vi "slow_control_2_14.vi"() -> ()   [LabVIEW 2018]
uses:
  4623b864-5764-45c6-9cb2-3e18237880ca.vi
  fa57f61f-0bb9-49ac-92eb-fcb40add4dbb.vi
  499f9cf5-7b15-41ea-951a-8da9be12721d.vi
  <vilib>/DAQmx/read.llb/DAQmx Read (Analog 1D DBL NChan 1Samp).vi
  ffb0d1b3-ef19-4e2e-b36e-7277177ef4b3.vi
  9a1acc8a-69db-4048-9e4c-bb07d66d2422.vi
  <vilib>/DAQmx/create/channels.llb/DAQmx Create Channel (AI-Voltage-Basic).vi
  <vilib>/DAQmx/create/channels.llb/DAQmx Create Channel (AI-Current-Basic).vi
  <vilib>/DAQmx/create/channels.llb/DAQmx Create Channel (AI-Temperature-RTD).vi
  <vilib>/DAQmx/miscellaneous.llb/DAQmx Fill In Error Info.vi
  <vilib>/Utility/file.llb/Read Delimited Spreadsheet (string).vi
  <instrlib>/Lake Shore 335/Lake Shore 335.lvlib
  <instrlib>/CAEN PSM/CAEN PSM.lvlib
  <resource>/objmgr/daqmx.rc
panel:
  out "Heater":dbl
  out "Coldhead":dbl
  out "Cycle number":i32
  out "Alarm state":bool
  out "Timestamp last \nmeasured (UPS)":timestamp
  out "Auto-clear":bool
  in  "Auto-clear data?":bool
  in  "Clear data":bool
  in  "Clear data every N cycles":dbl
  in  "N samples":i32=30
  out "Average Flow (SLPM)":dbl caption="Flow (SLPM)"
  out "CAEN Ch. Names":string[](array[string])
  in  "Cycles to execute":dbl=5.0 format="%#_13g"
  out "Detector Pressure":dbl
  in  "N samples":i32=20
  in  "Allows tabs on \nfront panel":T1(tab)
  in  "Specify up to six temperature sensors inside \nthe detector, separated with a comma.\nNumbers only, single commas!":string="10,11,12,13,14,15"
  out "Valid example:":string="11,12, 13, 15 ,14 "
  in  "Anode ch.":enum16{"1", "2", "3", "4"}(ring)=enum."3"
  in  "CAEN unit selector":enum16{"CAEN 1", "CAEN 2"}(ring)
  in  "Multipliers":dbl[](array[numeric])=[1.0, 1.0, 1.0, 1.0, 1.0, 1.0, 1.0, 1.0]
  in  "Offsets\nsubtracted":dbl[](array[numeric])=[0.0, 0.0, 0.0, 0.0, 0.0, 0.0, 0.0, 0.0]
  in  "Channel Names (9207, ai8:15)":string[](array[string])=["i0", "i1", "i2", "i3", "i4", "i5", "i6", "i7"] caption="\"Other\""
  in  "Flow meter input:":u16(ring)=3 items=["v0", "v1", "v2", "v3", "v4", "v5", "v6", "v7"]
  in  "Detector pressure input:":u16(ring) items=["v0", "v1", "v2", "v3", "v4", "v5", "v6", "v7"]
  in  "Channel Names (9207, ai0:7)":string[](array[string])=["v0", "v1", "v2", "v3", "v4", "v5", "v6", "v7"] caption="\"Other\""
  in  "Multipliers":dbl[](array[numeric])=[1.0, 1.0, 1.0, 1.0, 1.0, 1.0, 1.0, 1.0]
  in  "Offsets\nsubtracted":dbl[](array[numeric])=[0.0, 0.0, 0.0, 0.0, 0.0, 0.0, 0.0, 0.0]
  in  "Voltage channels":tag[](array[tag])=["9207/ai0", "9207/ai1", "9207/ai2", "9207/ai3", "9207/ai4", "9207/ai5", "9207/ai6", "9207/ai7"]
  in  "COM-port CAEN 1":refnum<visa-resource-name>
  in  "COM-port CAEN 2":refnum<visa-resource-name>
  in  "Run lakeshore?":bool
  in  "ID Query":bool
  in  "COM-port LakeShore":refnum<visa-resource-name>
  in  "PID settings":cluster{"P":dbl, "I":dbl, "D":dbl}={"P"=50.0, "I"=20.0, "D"=120.0}
  in  "Setpoint (°C)":dbl=-100.0 format="%.1f"
  in  "Heater range":u16(ring) items=["Off", "Low (On)", "Medium", "High"]
  in  "Current channels":tag[](array[tag])=["9207/ai8", "9207/ai9", "9207/ai10", "9207/ai11", "9207/ai12", "9207/ai13", "9207/ai14", "9207/ai15"]
  in  "Channel Names (CAEN)":string[](array[string])=["PMT 1", "PMT 2", "Anode", "Cathode", "Top gate", "Bottom gate", "Other 1", "Other 2"]
  in  "RTD Type":i32(ring)=10071 items=["Pt3750"=12481, "Pt3851"=10071, "Pt3911"=12482, "Pt3916"=10069, "Pt3920"=10053, "Pt3928"=12483, "Custom"=10137]
  in  "Module 1 channels (slot 1)":tag[](array[tag])=["cDAQ2Mod2/ai0", "cDAQ2Mod2/ai1", "cDAQ2Mod2/ai2", "cDAQ2Mod2/ai3", "cDAQ2Mod2/ai4", "cDAQ2Mod2/ai5", "cDAQ2Mod2/ai6", "cDAQ2Mod2/ai7"]
  in  "Current Excitation Source":i32(ring)=10200 items=["Internal"=10200, "External"=10167, "None"=10230]
  in  "Resistance Configuration":i32(ring)=3 items=["2-Wire"=2, "3-Wire"=3, "4-Wire"=4]
  in  "R (T = 0°C):":dbl=100.0
  in  "B":dbl
  in  "A":dbl
  in  "C":dbl
  in  "Module 2 channels (slot 2)":tag[](array[tag])=["cDAQ2Mod3/ai0", "cDAQ2Mod3/ai1", "cDAQ2Mod3/ai2", "cDAQ2Mod3/ai3", "cDAQ2Mod3/ai4", "cDAQ2Mod3/ai5", "cDAQ2Mod3/ai6", "cDAQ2Mod3/ai7"]
  in  "Shut off heater \nif Alarm is active":bool=TRUE
  in  "Re-save headers":bool
  in  "Resistance Configuration":i32(ring)=2 items=["2-Wire"=2, "3-Wire"=3, "4-Wire"=4]
  in  "Module 3 channels":tag[](array[tag])
  in  "RTD Type":i32(ring)=12481 items=["Pt3750"=12481, "Pt3851"=10071, "Pt3911"=12482, "Pt3916"=10069, "Pt3920"=10053, "Pt3928"=12483, "Custom"=10137]
  in  "R (T = 0°C)":dbl=100.0 format="%0.2f"
  out "PT1000 data":dbl[](array[numeric]) format="%0.2f"
  out "Det. T.":i32[](array[numeric])
  out "9207 (V; A) Converted":dbl[](array[numeric])
  out "9216 #1 (°C)":dbl[](array[numeric])
  out "9216 #2 (°C)":dbl[](array[numeric])
  out "Raw readouts (V, mA)":dbl[](array[numeric]) format="%0.2f"
  out "Det.P input #":i32
  out "Flow input #":i32
  out "PT100 data":dbl[](array[numeric]) format="%0.2f"
  in  "\"Sound\" alarm":bool
  in  "Sound alarm\nFrequency (Hz)":dbl=1680.0
  in  "Send status email now":bool
  out "Email error":i32
  out "source":string
  in  "Number of Bonus lines":i32=1
  out "Names (optional)":string[](array[string])
  in  "Send daily email?":bool=TRUE
  in  "Phone numbers":string[](array[string])
  out "Alarm (or test) message":string
  in  "Alarm\nMaster switch":bool
  in  "Repeat Alarm SMS\nevery N minutes":dbl=15.0
  in  "Test alarm":bool
  out "Warning":bool
  in  "UPS":bool
  in  "UPS Voltage \nLower Threshold":dbl=220.0
  out "String 6":string
  out "String 5":string
  out "String 4":string
  out "String 3":string
  out "String 2":string
  out "String":string
  out "NI mod 2&3 status":bool
  in  "NI mod 2&3":bool
  in  "NI mod 1":bool
  in  "CAEN 2":bool
  in  "CAEN 1":bool
  in  "LakeShore":bool
  out "Det. P. warning":bool
  out "Boolean 6":bool
  out "Boolean 5":bool
  out "Boolean 4":bool
  out "Boolean 3":bool
  out "Boolean 2":bool
  out "Boolean":bool
  in  "T 6":bool
  in  "T 5":bool
  in  "T 4":bool
  in  "T 3":bool
  in  "T 2":bool
  in  "T 1":bool
  in  "Detector Pressure":bool
  in  "Overpressure threshold":dbl
  in  "Underpressure threshold":dbl
  out "Comm. status":bool
  in  "High Temp threshold":dbl format="%#_13g"
  in  "Low Temp threshold":dbl format="%#_13g"
  out "LakeShore status":bool
  out "NI mod1 (P) status":bool
  out "CAEN 1 status":bool
  out "CAEN 2 status":bool
  out "Initialization status":bool
  out "Minimum input voltage measured":dbl
  out "Alarm active 2":bool
  out "SMS error":string
  out "Status email preview":string
  in  "Send status email at time:":string="14:00"
  in  "Email Addresses":string[](array[string])
  in  "return address":string="xamsups@gmail.com"
  in  "Ignore Initialization Errors":bool=TRUE caption="Ignore init. errors?"
  out "NI 9226":errorcluster
  in  "HV Channel status":string="Click the button to request the latest High Voltage channel status."
  out "CAEN 1":T2(array[cluster])
  out "CAEN 2":T2(array[cluster])
  in  "Query HV status":bool
  in  "\"code\"":string
  in  "String 7":string
  out "\"status\"":bool
  in  "\"source\"":string
  out "NI 9216 x2":errorcluster
  out "CAEN 1":errorcluster
  out "CAEN 2":errorcluster
  out "Lakeshore":errorcluster
  out "NI 9207":errorcluster
  out "9207 (ai 8:15, Amperes)":cluster{timestamp[], dbl[]}[](graph)
  in  "Temperature channel selector":u16(ring)=10 items=["10"=10, "11"=11, "12"=12, "13"=13, "14"=14, "15"=15, "Average"=666]
  out "Heater power (%)":cluster{timestamp[], dbl[]}[](graph)
  out "Flow (SLPM)":cluster{timestamp[], dbl[]}[](graph)
  out "9207 (ai 0:7, Volts)":cluster{timestamp[], dbl[]}[](graph)
  out "Phase Diagram":cluster{"X":dbl, "Y":dbl}[](graph)
  out "Temperature (ai 0:15, °C)":cluster{timestamp[], dbl[]}[](graph)
  in  "Pause?":bool
  out "Integrated Flow (SL)":dbl
  in  "Reset?":bool
  out "LakeShore readings":dbl[](array[numeric])
  out "Temp A":dbl
  out "Temp B":dbl
  in  "Temperature Channel Selector":u16(ring) items=["10"=10, "11"=11, "12"=12, "13"=13, "14"=14, "15"=15]
  out "Historical Large Phase Diagram":cluster{dbl[], dbl[]}[](graph)
  out "Large Phase Diagram":cluster{"X":dbl, "Y":dbl}[](graph)
  in  "Temperature Channel Selector":u16(ring)=666 items=["10"=10, "11"=11, "12"=12, "13"=13, "14"=14, "15"=15, "Average"=666]
  in  "Scale.Range:Minimum 8":dbl
  in  "Scale.Range:Maximum 8":dbl=4000.0
  in  "Scale.Range:Minimum 7":dbl
  in  "Scale.Range:Maximum 7":dbl=4000.0
  in  "Scale.Range:Minimum 6":dbl=-3000.0
  in  "Scale.Range:Maximum 6":dbl
  in  "Scale.Range:Minimum 5":dbl
  in  "Scale.Range:Maximum 5":dbl=3000.0
  in  "Scale.Range:Minimum 4":dbl=-5000.0
  in  "Scale.Range:Maximum 4":dbl
  in  "Scale.Range:Maximum 3":dbl=4000.0
  in  "Scale.Range:Minimum 3":dbl
  in  "Scale.Range:Maximum 2":dbl=1000.0
  in  "Scale.Range:Minimum 2":dbl
  out "CAEN 1.1":dbl(knob) scale=0.0..1000.0
  out "CAEN 1.1":string
  in  "Scale.Range:Maximum":dbl=1000.0
  in  "Scale.Range:Minimum":dbl
  out "CAEN 2.3 2":string
  out "CAEN 2.2 2":string
  out "Channel Names":string[](array[string])
  out "CAEN 2.3":dbl(knob) scale=0.0..4000.0
  out "CAEN 2.2":dbl(knob) scale=0.0..4000.0
  out "CAEN 2.1":string
  out "CAEN 2.0":string
  out "CAEN 1.3":string
  out "CAEN 1.2":string
  out "CAEN 1.0":string
  out "Channel Names":string[](array[string])
  in  "Set to zero":bool
  out "CAEN 2.1":dbl(knob)
  out "CAEN 2.0":dbl(knob) scale=0.0..3000.0
  in  "Apply Voltage":bool
  in  "VSet (V)":dbl[](array[numeric])
  in  "IMax (uA)":dbl[](array[numeric])
  in  "VMax (V)":dbl[](array[numeric])
  out "CAEN 1.3":dbl(knob)
  out "CAEN 1.2":dbl(knob) scale=0.0..4000.0
  out "CAEN 1.0":dbl(knob) scale=0.0..1000.0
  out "Vmon (V)":dbl[](array[numeric])
  out "IMon (uA)":dbl[](array[numeric])
  in  "Read CAEN units \nevery N cycles":i16=120
  in  "Reset anode\nperiodically?":bool
  in  "Kill every Y minutes":i32=10
  in  "Keep off for X seconds":i32=10
  out "?":bool
  out "Killed":bool
  out "Restarted":bool
  out "Anode timers":timestamp[](array[timestamp])
  out "Seconds until \nanode autokill":dbl format="%.2g"
  out "Seconds until \nanode reset":dbl format="%.2g"
  in  "Kill voltage":bool
  in  "stop":bool
  out "Voltages":dbl[](array[numeric])
  out "Started up?":bool
  out "TOBA appended":dbl[][](array[numeric])
  in  "Read T every N cycles":i32=2
  out "Time until next cycle":dbl format="%.3g"
  in  "Time per cycle (s)":i32=2 caption="Time Target (s)"
  # "<- Proof of concept for New/Old T + New P"
  # "Moving averages"
  # "NI 9216 Temperature settings"
  # "CAEN settings"
  # "NI 9207 Voltage settings"
  # "If RTD type is custom,\nspecify the Callendar-\nVan Dusen parameters"
  # "Anode connected to:"
  # "Channel:"
  # "NI 9207 Current settings"
  # "Lakeshore settings"
  # "NI 9226 Temperature settings"
  # "Gain (P) (XX.X)"
  # "Reset (I) (XX.X)"
  # "Rate (D) (X.X%)"
  # "Alarm indicators and arms"
  # "Detector Thresholds"
  # "Daily status email"
  # "SMS and sound alarm"
  # "Alarm conditions"
  # "Temperature channels:"
  # "Uninterruptable Power Supply"
  # "Device information"
  # "High Voltage channel status"
  # "How-to"
  # "Data"
  # "Scale:"
  # "to"
  # "to"
  # "Scale:"
  # "Time of last reset"
  # "Time of last reactivation"
  # "to"
  # "Scale:"
  # "to"
  # "Scale:"
  # "Settings"
  # "Scale:"
  # "to"
  # "Scale:"
  # "to"
  # "Scale:"
  # "to"
  # "to"
  # "Scale:"
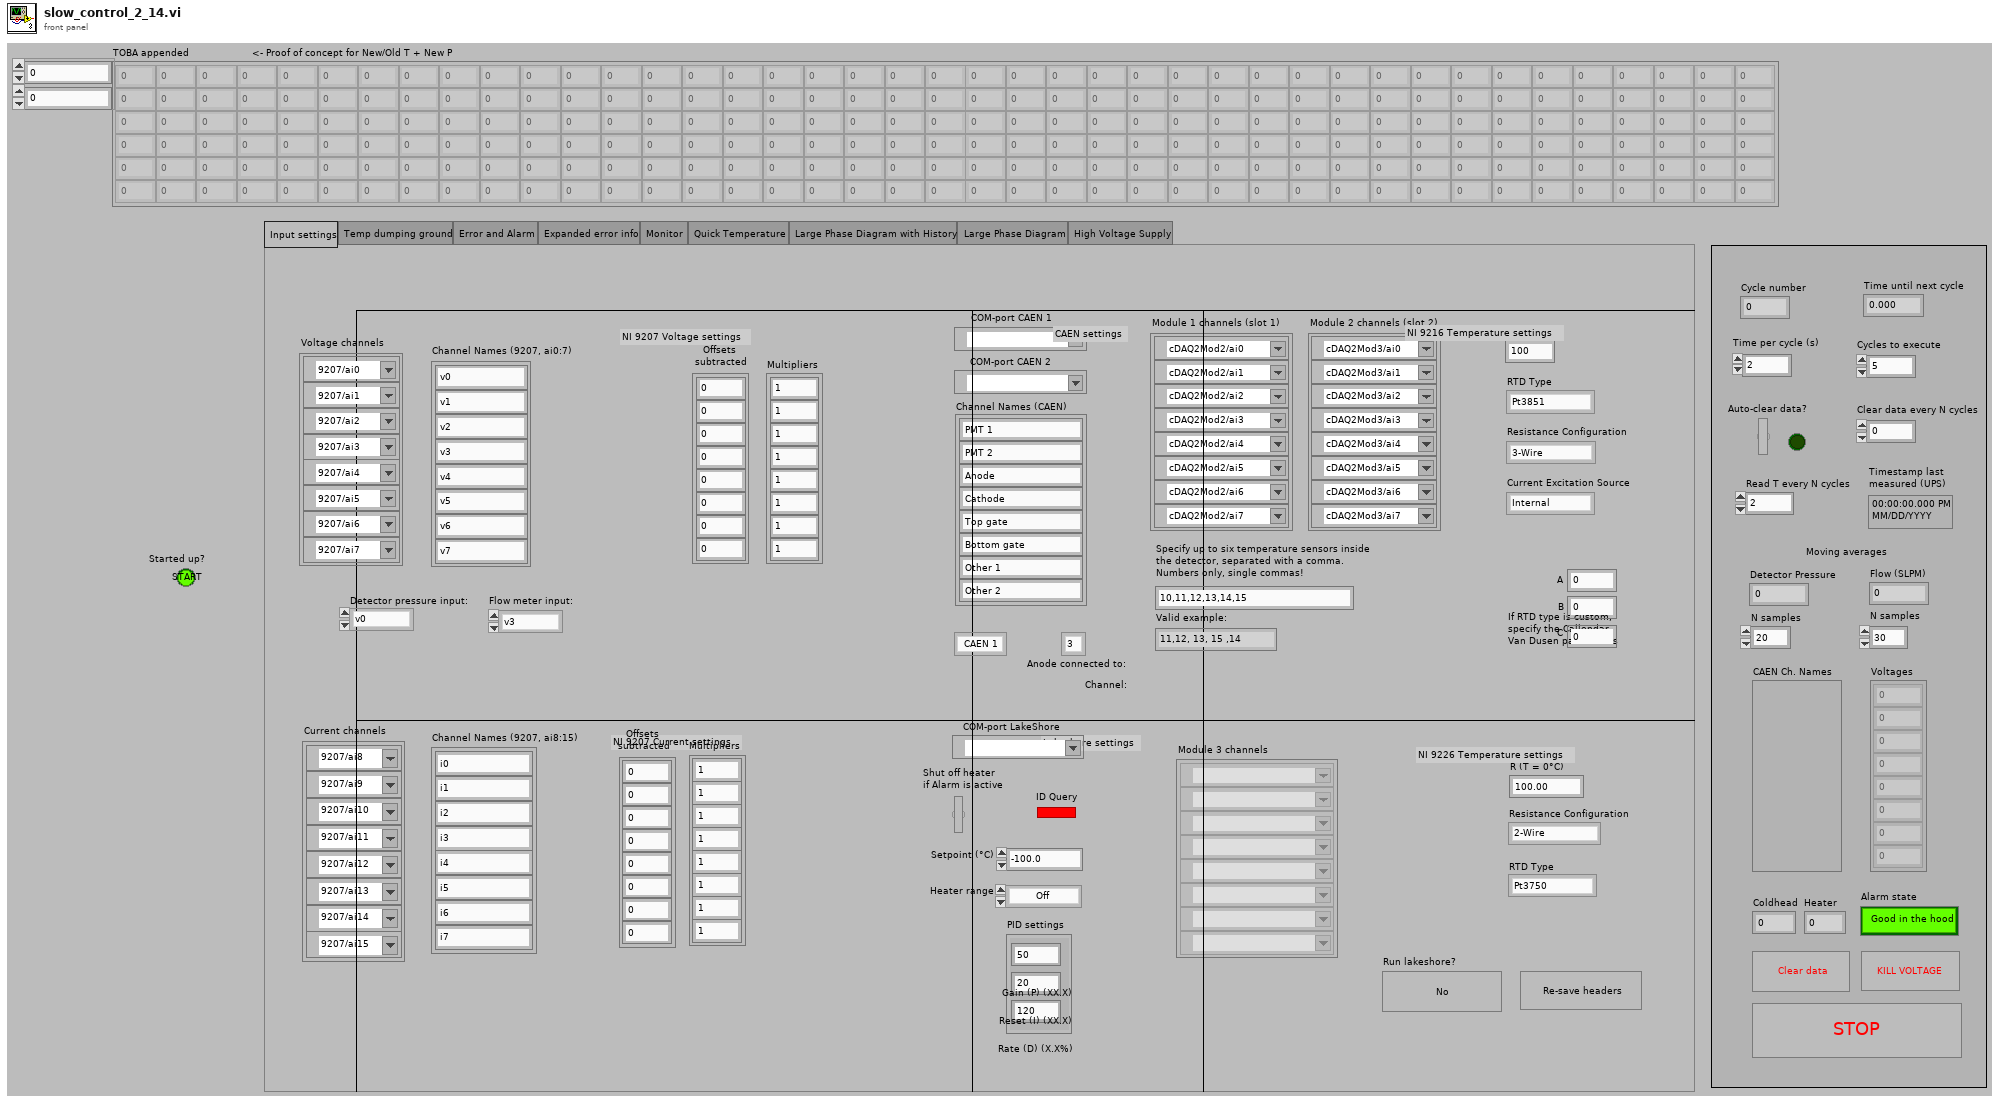
[diagram p1: front panel]
types:
  T1 = enum32{"Input settings", "Temp dumping ground", "Error and Alarm", "Expanded error info", "Monitor", "Quick Temperature", "Large Phase Diagram with History", "Large Phase Diagram", "High Voltage Supply"}
  T2 = cluster{"ON":bool, "RUP":bool, "RDW":bool, "OVC":bool, "OVV":bool, "UNV":bool, "MAXV":bool, "TRIP":bool, "OVP":bool, "OVT":bool, "DIS":bool, "KILL":bool, "ILK":bool, "NOCAL":bool}[]
  T3 = cluster{"Baud Rate":u32, "Parity":u16, "Data Bits":u16, "Stop Bits":u16, "Flow Control":u16}
  T4 = cluster{"task out":refnum<k21>, "error out":errorcluster}
  T5 = cluster{"VISA resource name out":refnum<visa-resource-name>, "error out":errorcluster}
  T6 = cluster{"VISA resource name out":refnum<visa-resource-name>, "Board address":u8, "NChannels":u8}
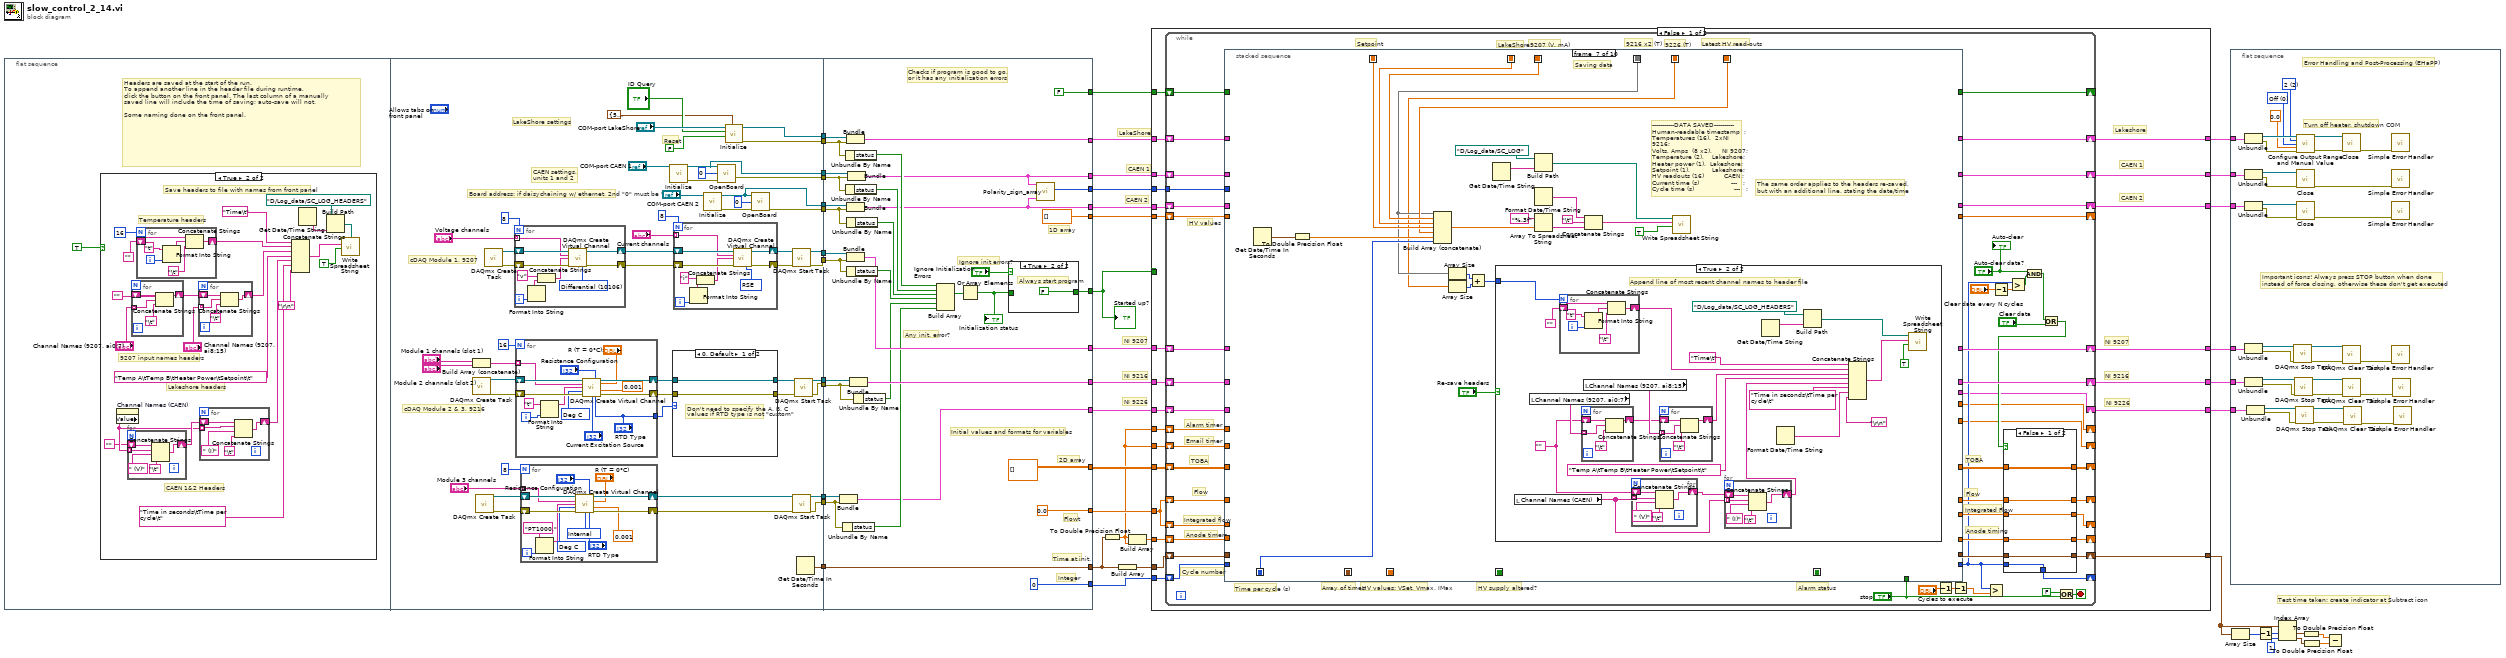
[diagram p0: block diagram]
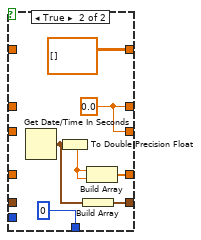
[diagram p2: hidden frame]
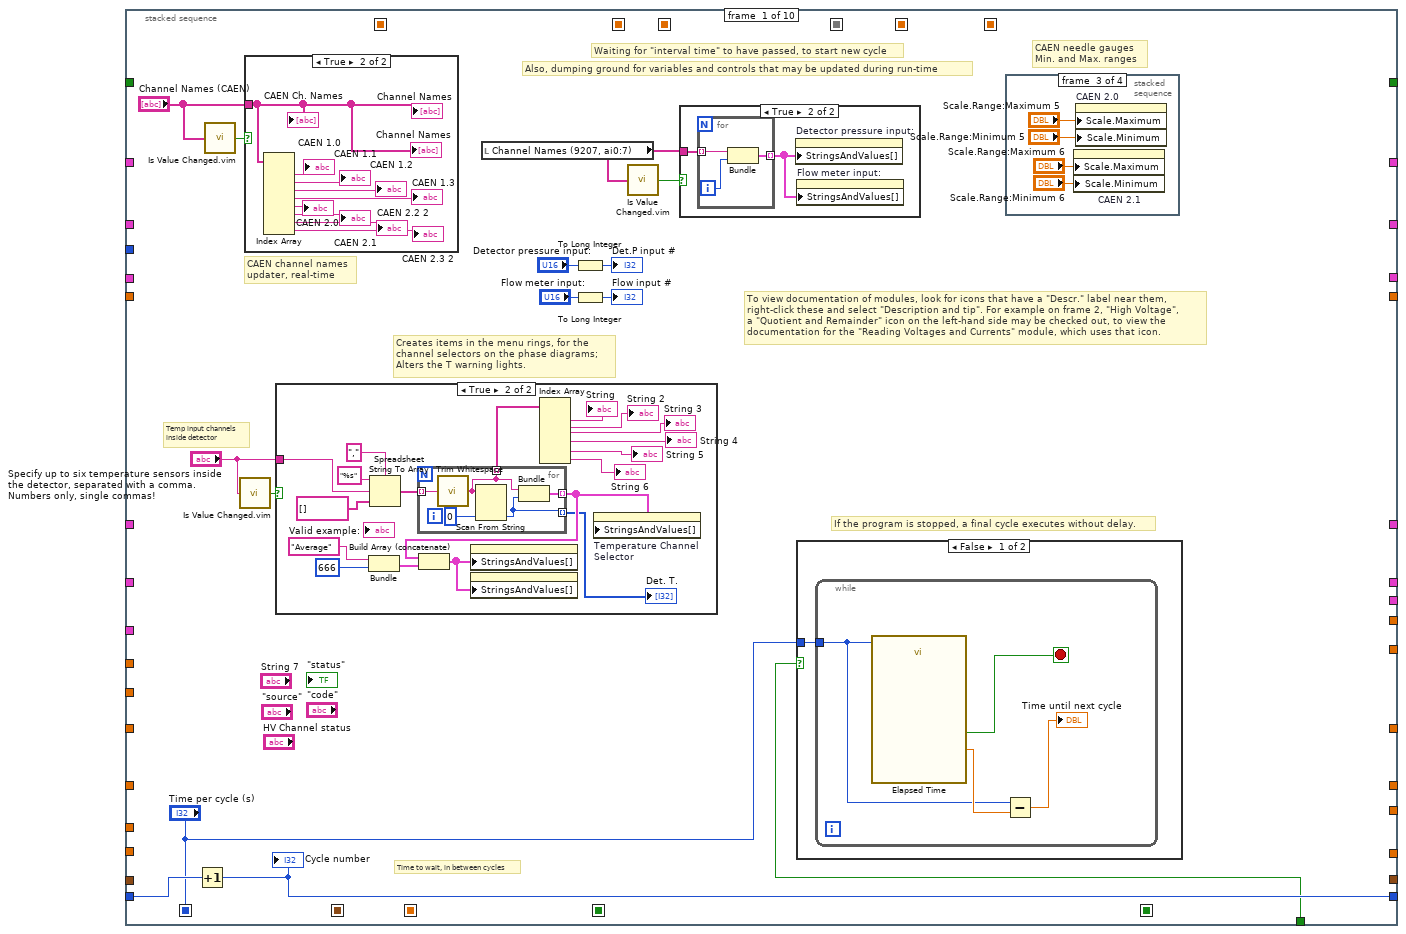
[diagram p3: hidden frame]
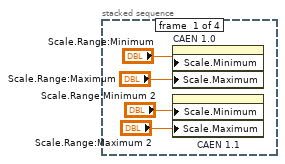
[diagram p7: hidden frame]
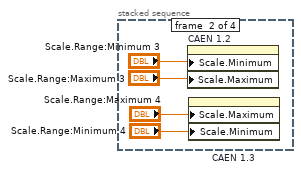
[diagram p8: hidden frame]
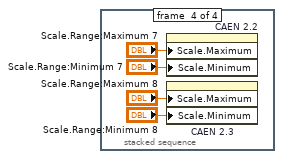
[diagram p9: hidden frame]
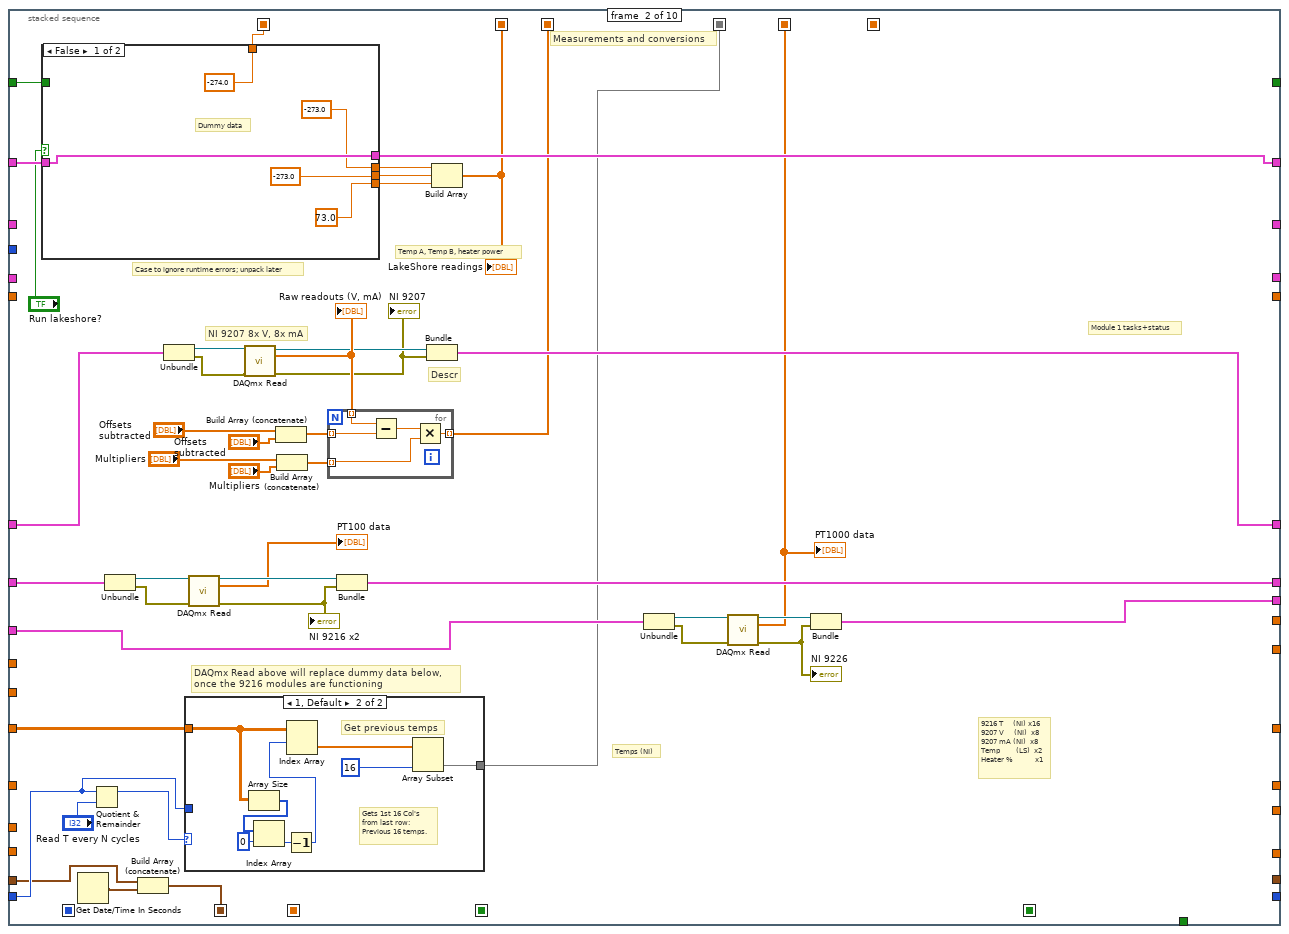
[diagram p11: hidden frame]
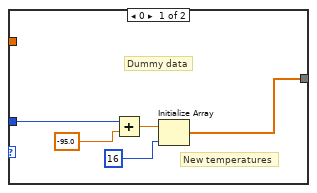
[diagram p12: hidden frame]
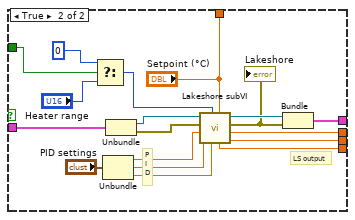
[diagram p13: hidden frame]
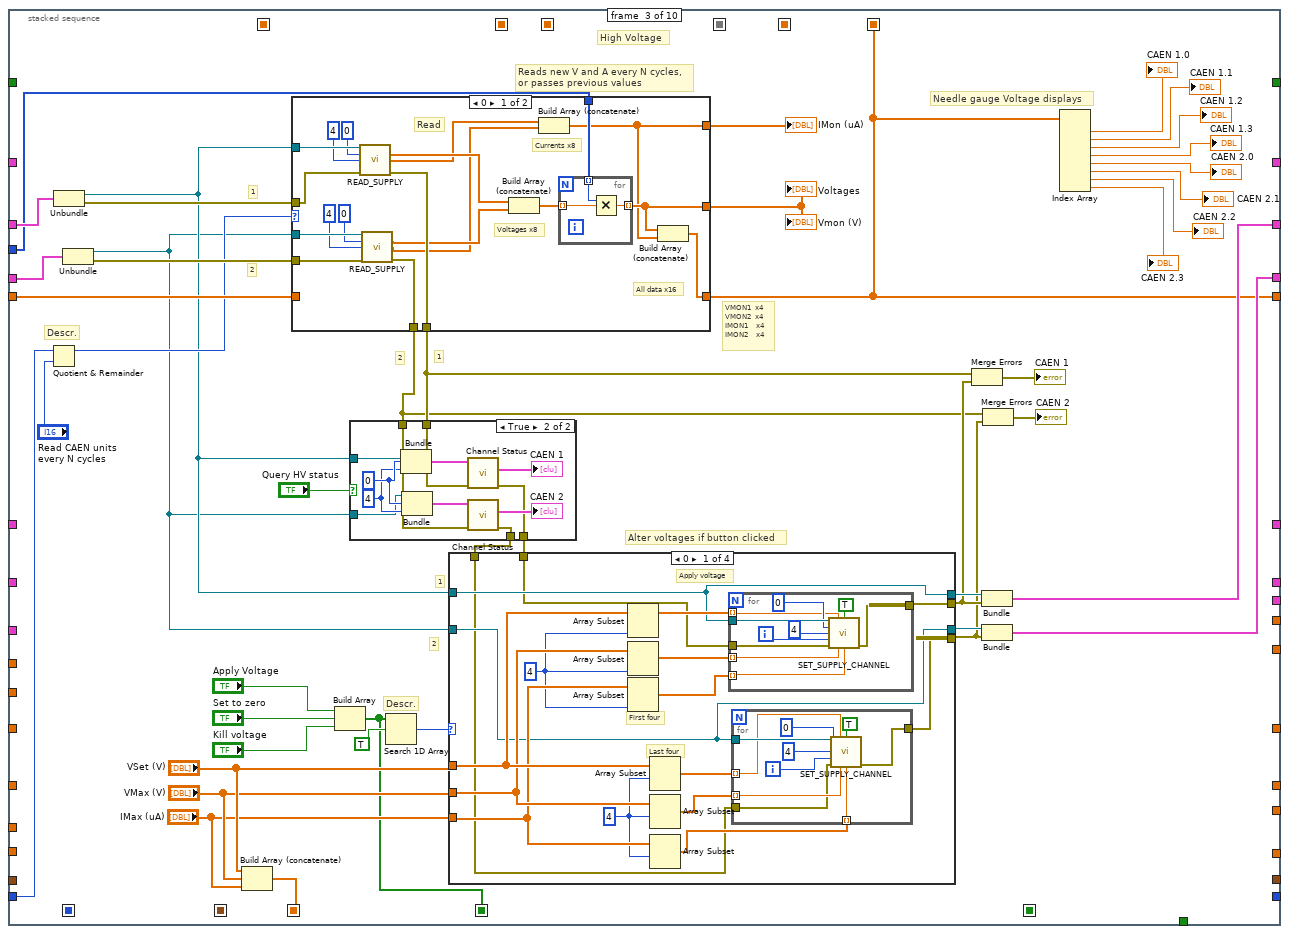
[diagram p14: hidden frame]
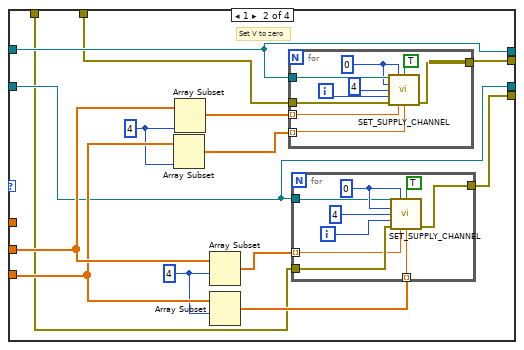
[diagram p16: hidden frame]
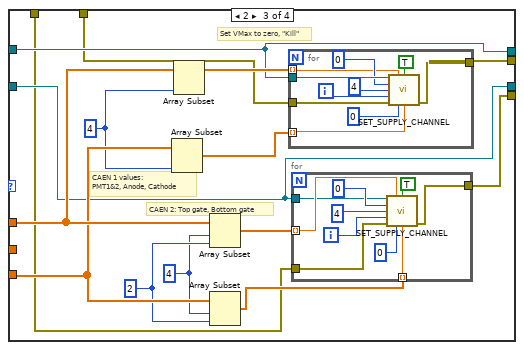
[diagram p17: hidden frame]
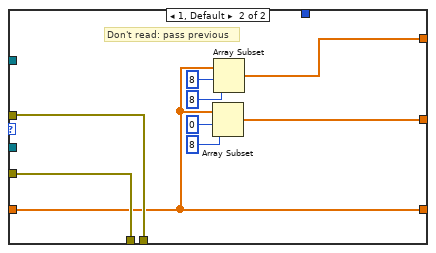
[diagram p19: hidden frame]
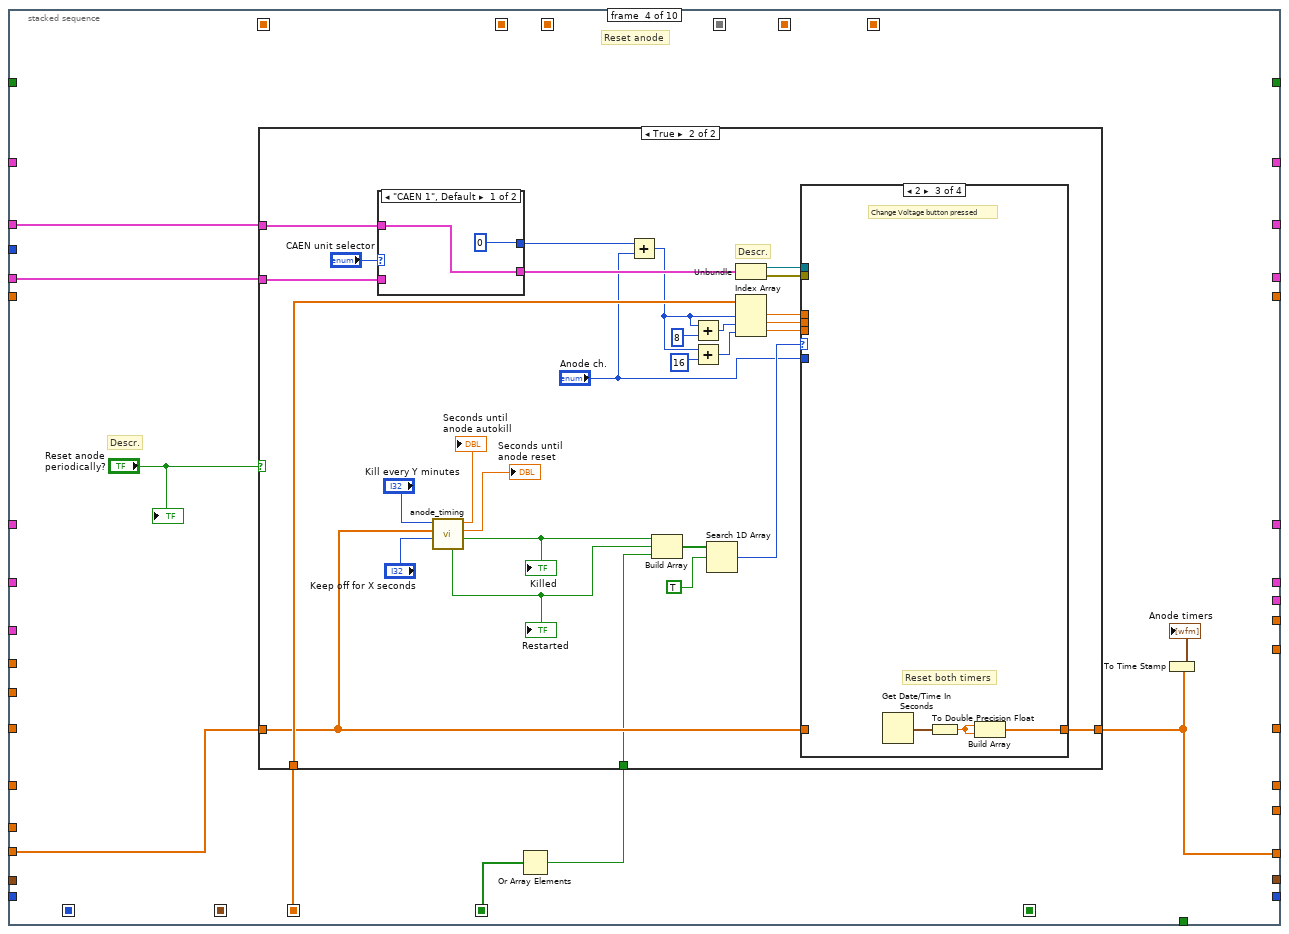
[diagram p20: hidden frame]
diagram:
  # "NI 9226"
  # "NI 9216"
  # "Test time taken: create indicator at Subtract icon"
  # "NI 9207"
  # "CAEN 2"
  # "CAEN 1"
  # "LakeShore"
  n1 = flat-sequence {
    tunnel: [w137] -> w44
    tunnel: [w136] -> w43
    tunnel: [w124] -> w42
    tunnel: [w133] -> w41
    tunnel: [w114] -> w40
    tunnel: [w132] -> w35
    tunnel: [w128] -> w27
    tunnel: [w127] -> w26
    tunnel: [w115] -> w18
    tunnel: [w109] -> w10
    tunnel: [w108] -> w9
    tunnel: [w92] -> w5
    tunnel: [w91] -> w4
    tunnel: w44 -> [w229]
    tunnel: w43 -> [w228]
    tunnel: w42 -> [w226]
    tunnel: w41 -> [w225]
    tunnel: w40 -> [w217]
    tunnel: [w230] -> w24
    tunnel: [0.0] -> w23
    tunnel: [dbl[] []] -> w39
    tunnel: [dbl[][] []] -> w11
    tunnel: [0] -> w38
    tunnel: [w227] -> w37
    tunnel: [w200] -> w36
    tunnel: [w224] -> w22
    tunnel: w35 -> [w224]
    tunnel: w27 -> [w222]
    tunnel: w26 -> [w221]
    tunnel: [w199] -> w25
    tunnel: [FALSE] -> w19
    tunnel: w18 -> [w218]
    tunnel: [w216] -> w17
    tunnel: w10 -> [w209]
    tunnel: w9 -> [w208]
    tunnel: [w207] -> w8
    tunnel: w5 -> [w204]
    tunnel: w4 -> [w203]
    tunnel: [w201] -> w3
    tunnel: [w198] -> w1
    frame #0 {
      # "Headers are saved at the start of the run.\nTo append another line in the header file during runtime,\nclick the button on the front panel. The last column of a manually\nsaved line will include the time of saving; auto-save will not.\n\nSome naming done on the front panel."
      n2 = case shown="True" TRUE {
        frame False {
        }
        frame True {
          # "CAEN 1&2 Headers"
          # "Lakeshore headers"
          # "9207 input names headers"
          # "Temperature headers"
          # "Save headers to file with names from front panel"
          n3 = property on="Channel Names (CAEN)" class="Arr (strict)"() -> ("Value"=w51:string[])  [unwired: 2 in, 2 out]
          n4 = for {
            tunnel: w51 -> [w75] mode=indexing
            shift-right: [w73] -> w52
            shift-left: "" -> [w72]
            n5 = Concatenate Strings(w72, w75, " (V)", "\t") -> (w73:string)
          }
          n6 = for {
            shift-right: [w83] -> w55
            shift-left: "" -> [w84]
            tunnel: "Channel Names (9207, ai0:7)" -> [w81] mode=indexing
            n7 = Concatenate Strings(w84, w81, "\t") -> (w83:string)
          }
          n8 = for {
            N: 16 -> [_]
            shift-right: [w85] -> w58
            shift-left: "" -> [w86]
            i -> [w90]
            n9 = Format Into String(initial string="t", w90) -> (resulting string=w88:string)  [unwired: 2 in, 1 out]
            n10 = Concatenate Strings(w86, w88, "\t") -> (w85:string)
          }
          n11 = for {
            shift-right: [w78] -> w54
            shift-left: w55 -> [w80]
            tunnel: "Channel Names (9207, ai8:15)" -> [w77] mode=indexing
            n12 = Concatenate Strings(w80, w77, "\t") -> (w78:string)
          }
          n13 = for {
            shift-right: [w68] -> w50
            shift-left: w52 -> [w69]
            tunnel: w51 -> [w67] mode=indexing
            n14 = Concatenate Strings(w69, w67, " (I)", "\t") -> (w68:string)
          }
          n15 = Concatenate Strings("Time\t", w58, w54, "Temp A\tTemp B\tHeater Power\tSetpoint\t", w50, "Time in seconds\tTime per cycle\t", "\r\n") -> (w57:string)
          n16 = Get Date/Time String() -> (date string=w61:string)  [unwired: 3 in, 1 out]
          n17 = Build Path(base path=path "D:/Log_data/SC_LOG_HEADERS" ("file path (dialog if empty)"), name or relative path=w61) -> (appended path=w62:path)
          n18 = call <vilib>:"Write Spreadsheet String.vi"("append to file? (new file:F)"=TRUE, "spreadsheet string"=w57, "file path (dialog if empty)"=w62) -> ()  [unwired: 7 in, 2 out]
        }
      }
    }
    frame #1 {
      # "cDAQ Module 2 & 3, 9216"
      # "cDAQ Module 1, 9207"
      # "Board address: if daisychaining w/ ethernet, 2nd \"0\" must be \"1\""
      # "CAEN settings,\nunits 1 and 2"
      # "Reset"
      # "LakeShore settings"
      n19 = call <vilib>:"DAQmx Create Task.vi"() -> ("task out"=w107:refnum<k21>, "error out"=w110:errorcluster)  [unwired: 14 in]
      n20 = Build Array (concatenate)("Module 1 channels (slot 1)", "Module 2 channels (slot 2)") -> (w104:tag[])
      n21 = call <vilib>:"DAQmx Create Task.vi"() -> ("task out"=w97:refnum<k21>, "error out"=w96:errorcluster)  [unwired: 14 in]
      n22 = call <vilib>:"DAQmx Create Task.vi"() -> ("task out"=w123:refnum<k21>, "error out"=w122:errorcluster)  [unwired: 14 in]
      n23 = for {
        N: 8 -> [_]
        shift-right: [w193] -> w119
        shift-left: w123 -> [w192]
        shift-right: [w194] -> w118
        shift-left: w122 -> [w190]
        tunnel: "Voltage channels" -> [w191] mode=indexing
        i -> [w196]
        w188 = 10106 items=["Default"=-1, "RSE"=10083, "NRSE"=10078, "Differential"=10106, "Pseudodifferential"=12529] ("input terminal configuration")
        n24 = Format Into String(w196) -> (resulting string=w195:string)  [unwired: 3 in, 1 out]
        n25 = Concatenate Strings("v" ("string"), w195) -> (w189:string)
        n26 = call-poly <vilib>:"DAQmx Create Virtual Channel.vi"("task in"=w192, "input terminal configuration"=w188, "physical channels"=w191, "name to assign"=w189, "error in"=w190) -> ("task out"=w193:refnum<k21>, "error out"=w194:errorcluster)  [unwired: 9 in]
      }
      n27 = for {
        N: 16 -> [_]
        shift-right: [w174] -> w103
        shift-left: w107 -> [w177]
        shift-right: [w175] -> w102
        shift-left: w110 -> [w176]
        tunnel: w104 -> [w173] mode=indexing
        tunnel: ["RTD Type"] -> w99
        i -> [w171]
        w168 = 10143 items=["Deg C"=10143, "Deg F"=10144, "Kelvins"=10325, "Deg R"=10145, "From Custom Scale"=10065] ("units")
        n28 = Format Into String(initial string="t", w171) -> (resulting string=w170:string)  [unwired: 2 in, 1 out]
        n29 = call-poly <vilib>:"DAQmx Create Virtual Channel.vi"("task in"=w177, "resistance configuration"="Resistance Configuration", "physical channels"=w173, "r0"="R (T = 0°C):", "name to assign"=w170, "units"=w168, "current excitation value"=0.001, "error in"=w176, "current excitation source"="Current Excitation Source", "rtd type"="RTD Type") -> ("task out"=w174:refnum<k21>, "error out"=w175:errorcluster)  [unwired: 4 in]
      }
      n30 = for {
        N: 8 -> [_]
        shift-right: [w152] -> w94
        shift-left: w97 -> [w151]
        shift-right: [w153] -> w93
        shift-left: w96 -> [w154]
        tunnel: "Module 3 channels" -> [w149] mode=indexing
        i -> [w147]
        w143 = 10200 items=["Internal"=10200, "External"=10167, "None"=10230] ("current excitation source")
        w145 = 10143 items=["Deg C"=10143, "Deg F"=10144, "Kelvins"=10325, "Deg R"=10145, "From Custom Scale"=10065] ("units")
        n31 = Format Into String(initial string="PT1000.", w147) -> (resulting string=w146:string)  [unwired: 2 in, 1 out]
        n32 = call-poly <vilib>:"DAQmx Create Virtual Channel.vi"("task in"=w151, "resistance configuration"="Resistance Configuration", "physical channels"=w149, "r0"="R (T = 0°C)", "name to assign"=w146, "units"=w145, "current excitation value"=0.001, "error in"=w154, "current excitation source"=w143, "rtd type"="RTD Type") -> ("task out"=w152:refnum<k21>, "error out"=w153:errorcluster)  [unwired: 4 in]
      }
      n33 = call <instrlib>:"Initialize.vi"("VISA resource name"="COM-port CAEN 1") -> ("error out"=w134:errorcluster, "VISA resource name out"=w124:refnum<visa-resource-name>)  [unwired: 9 in]
      n34 = case shown="0, Default" w99 {
        tunnel: w103 -> [w156 w160]
        tunnel: w102 -> [w155 w159]
        tunnel: [w156 w158] -> w101
        tunnel: [w155 w157] -> w100
        frame 0, Default {
          # "Don't need to specify the A, B, C\nvalues if RTD type is not \"custom\""
        }
        frame 10137 {
          # "RTD type =  \"custom\""
          n35 = property class="DAQmx Channel"(reference=w160, error in=w159, "AI.RTD.A"="A", "AI.RTD.B"="B", "AI.RTD.C"="C") -> (reference out=w158:refnum<k21>, error out=w157:errorcluster)
        }
      }
      n36 = for {
        N: 8 -> [_]
        shift-right: [w179] -> w116
        shift-left: w119 -> [w186]
        shift-right: [w178] -> w117
        shift-left: w118 -> [w185]
        tunnel: "Current channels" -> [w184] mode=indexing
        i -> [w183]
        w187 = 10083 items=["default"=-1, "RSE"=10083, "NRSE"=10078, "Differential"=10106, "Pseudodifferential"=12529] ("input terminal configuration")
        n37 = Format Into String(w183) -> (resulting string=w181:string)  [unwired: 3 in, 1 out]
        n38 = Concatenate Strings("i", w181) -> (w180:string)
        n39 = call-poly <vilib>:"DAQmx Create Virtual Channel.vi"("task in"=w186, "input terminal configuration"=w187, "physical channels"=w184, "name to assign"=w180, "error in"=w185) -> ("task out"=w179:refnum<k21>, "error out"=w178:errorcluster)  [unwired: 9 in]
      }
      n40 = call <instrlib>:"Initialize.vi"("VISA resource name"="COM-port CAEN 2") -> ("error out"=w129:errorcluster, "VISA resource name out"=w128:refnum<visa-resource-name>)  [unwired: 9 in]
      n41 = call <instrlib>:"OpenBoard.vi"("error in (no error)"=w134, "Board Address"=0, "VISA resource name"=w124) -> ("error out"=w133:errorcluster)  [unwired: 7 in, 1 out]
      n42 = call <instrlib>:"Initialize.vi"("Serial Configuration"=T3 {"Baud Rate"=57600, "Parity"=1, "Data Bits"=7, "Stop Bits"=10, "Flow Control"=0}, "Reset (True)"=FALSE ("Reset (LakeShore)"), "ID Query (True)"="ID Query", "VISA resource name"="COM-port LakeShore") -> ("error out"=w136:errorcluster, "VISA resource name out"=w137:refnum<visa-resource-name>)  [unwired: 6 in]
      n43 = call <instrlib>:"OpenBoard.vi"("error in (no error)"=w129, "Board Address"=u8 0, "VISA resource name"=w128) -> ("error out"=w127:errorcluster)  [unwired: 7 in, 1 out]
      n44 = call <vilib>:"DAQmx Start Task.vi"("task/channels in"=w116, "error in"=w117) -> ("task out"=w115:refnum<k21>, "error out"=w114:errorcluster)  [unwired: 12 in]
      n45 = call <vilib>:"DAQmx Start Task.vi"("task/channels in"=w94, "error in"=w93) -> ("task out"=w92:refnum<k21>, "error out"=w91:errorcluster)  [unwired: 12 in]
      n46 = call <vilib>:"DAQmx Start Task.vi"("task/channels in"=w101, "error in"=w100) -> ("task out"=w109:refnum<k21>, "error out"=w108:errorcluster)  [unwired: 12 in]
      n47 = Get Date/Time In Seconds() -> (seconds since 1Jan1904=w132:timestamp)
    }
    frame #2 {
      # "1D array"
      # "Initial values and formats for variables"
      # "Time at init."
      # "Integer"
      # "2D array"
      # "Flowt"
      # "Checks if program is good to go,\nor it has any initialization errors"
      # "Ignore init errors?"
      # "Any init. error?"
      n48 = Bundle("task out"=w204, "error out"=w203) -> (w201:T4)  [unwired: 1 in]
      n49 = Unbundle By Name(w203) -> ("status"=w202:bool)
      n50 = Unbundle By Name(w225) -> ("status"=w231:bool)
      n51 = Unbundle By Name(w228) -> ("status"=w210:bool)
      n52 = Bundle("VISA resource name out"=w229, "error out"=w228) -> (w227:T5)  [unwired: 1 in]
      n53 = Unbundle By Name(w221) -> ("status"=w223:bool)
      n54 = Unbundle By Name(w217) -> ("status"=w211:bool)
      n55 = Bundle("VISA resource name out"=w222, "error out"=w221) -> (w199:T5)  [unwired: 1 in]
      n56 = Bundle("task out"=w218, "error out"=w217) -> (w216:T4)  [unwired: 1 in]
      n57 = Bundle("VISA resource name out"=w226, "error out"=w225) -> (w200:T5)  [unwired: 1 in]
      n58 = Bundle("task out"=w209, "error out"=w208) -> (w207:T4)  [unwired: 1 in]
      n59 = Unbundle By Name(w208) -> ("status"=w206:bool)
      n60 = Build Array(w210, w231, w211, w223, w206, w202) -> (w232:bool[])
      n61 = Or Array Elements(Boolean array=w232) -> (logical OR=w205:bool)
      "Initialization status" <- w205
      n62 = case shown="True" "Ignore Initialization Errors" {
        tunnel: [w233 FALSE] -> w230
        tunnel: w205 -> [w233 _]
        frame False {
          # "Only start if no errors"
        }
        frame True {
          # "Always start program"
        }
      }
      n63 = call "Polarity_sign_array.vi"("CAEN 2 in"=w199, "CAEN 1 in"=w200) -> ("Polarity signs"=w198:i32[])  [unwired: 7 in, 2 out]
    }
  }
  n64 = To Double Precision Float(number=w22) -> (double precision float=w6:dbl)
  n65 = Build Array(w22) -> (w34:timestamp[])
  n66 = Build Array(w6, w6) -> (w21:dbl[])
  n67 = case shown="False" w24 {
    selector: w24 -> [_ w1197]
    tunnel: [_ w1197] -> _
    tunnel: w39 -> [w250 _]
    tunnel: w38 -> [w257 _]
    tunnel: w11 -> [w256 _]
    tunnel: w37 -> [w251 w1195]
    tunnel: w36 -> [w253 w1194]
    tunnel: w34 -> [w255 _]
    tunnel: [w254 timestamp[] []] -> w30
    tunnel: w25 -> [w252 w1193]
    tunnel: w23 -> [w246 _]
    tunnel: w21 -> [w249 _]
    tunnel: [w248 w1195] -> w20
    tunnel: w19 -> [w247 _]
    tunnel: w17 -> [w245 w1192]
    tunnel: [w244 w1194] -> w16
    tunnel: [w243 w1193] -> w15
    tunnel: [w242 w1192] -> w14
    tunnel: w8 -> [w241 w1191]
    tunnel: [w240 w1191] -> w7
    tunnel: w6 -> [w239 _]
    tunnel: w6 -> [w238 _]
    tunnel: w3 -> [w237 w1190]
    tunnel: [w236 w1190] -> w2
    tunnel: w1 -> [w235 _]
    frame False {
      # "NI 9226"
      # "NI 9216"
      # "NI 9207"
      # "CAEN 2"
      # "CAEN 1"
      # "Lakeshore"
      n68 = while {
        shift-right: [w271] -> _
        shift-left: w257 -> [w309]
        shift-right: [w284] -> _
        shift-left: w256 -> [w298]
        shift-right: [w276] -> w254
        shift-left: w255 -> [w306]
        shift-right: [w300] -> w244
        shift-left: w253 -> [w293]
        shift-right: [w302] -> _
        shift-left: w250 -> [w305]
        shift-right: [w299] -> w243
        shift-left: w252 -> [w304]
        shift-right: [w301] -> w248
        shift-left: w251 -> [w303]
        shift-right: [w280] -> _
        shift-left: w246 -> [w295]
        shift-right: [w282] -> _
        shift-left: w246 -> [w296]
        shift-right: [w278] -> _
        shift-left: w249 -> [w294]
        shift-right: [w266] -> _
        shift-left: w247 -> [w292]
        shift-right: [w290] -> w242
        shift-left: w245 -> [w291]
        shift-right: [w288] -> w240
        shift-left: w241 -> [w289]
        shift-right: [w264] -> _
        shift-left: w239 -> [w265]
        shift-right: [w261] -> _
        shift-left: w238 -> [w262]
        shift-right: [w259] -> w236
        shift-left: w237 -> [w260]
        tunnel: w235 -> [w258]
        stop <- w307 stop-if-true
        # "9226 (T)"
        # "Email timer"
        # "Alarm timer"
        # "Alarm status"
        # "LakeShore"
        # "9216 x2 (T)"
        # "9207 (V, mA)"
        # "HV supply altered?"
        # "Setpoint"
        # "Anode timing"
        # "Anode timers"
        # "Integrated flow"
        # "Flow"
        # "Flow"
        # "Integrated Flow"
        # "TOBA"
        # "Array of times"
        # "Latest HV read-outs"
        # "Time per cycle (s)"
        # "Cycle number"
        # "HV values: VSet, Vmax, IMax"
        # "HV values"
        # "TOBA"
        n69 = stacked-sequence {
          seq-local: [_ _ w502 _ _ _ _ _ _ _] -> [_ _ _ w685 _ _ _ _ _ _]
          seq-local: ["Time per cycle (s)" _ _ _ _ _ _ _ _ _] -> [_ _ _ _ _ _ w889 _ _ _]
          seq-local: [_ _ w493 _ _ _ _ _ _ _] -> [_ _ _ _ _ _ w891 _ _ _]
          seq-local: [_ w435 _ _ _ _ _ _ _ _] -> [_ _ _ _ w760 w872 _ _ _ _]
          seq-local: [_ _ w496 _ _ _ _ _ _ _] -> [_ _ _ w680 _ _ _ _ _ _]
          seq-local: [_ w428 _ _ _ _ _ _ _ _] -> [_ _ _ _ _ _ w905 _ _ _]
          seq-local: [_ w423 _ _ _ _ _ _ _ _] -> [_ _ _ _ w767 w864 w893 w993 w1028 w1115]
          seq-local: [_ w395 _ _ _ _ _ _ _ _] -> [_ _ _ _ w772 w867 w885 w994 w1027 w1117]
          seq-local: [_ w411 _ _ _ _ _ _ _ _] -> [_ _ _ _ w771 w866 w892 _ _ _]
          seq-local: [_ _ _ _ _ _ _ w953 _ _] -> [_ _ _ _ _ _ _ _ w1030 w1116]
          seq-local: [_ w396 _ _ _ _ _ _ _ _] -> [_ _ _ _ w770 _ w884 _ _ _]
          tunnel: [w335 _ _ _ _ _ _ _ _ _] -> w270
          tunnel: "stop" -> [w334 _ _ _ _ _ _ _ _ _]
          tunnel: w309 -> [w336 w424 w518 _ _ _ _ _ _ _]
          tunnel: w298 -> [_ w425 _ _ w804 _ _ _ _ _]
          tunnel: [_ _ _ _ w758 _ _ _ _ _] -> w285
          tunnel: w306 -> [_ w403 _ _ _ _ _ _ _ _]
          tunnel: w293 -> [_ _ w525 w686 _ _ _ w1010 _ _]
          tunnel: w305 -> [_ _ w523 _ _ _ _ _ _ _]
          tunnel: w304 -> [_ _ w522 w681 _ _ _ w1009 _ _]
          tunnel: w303 -> [_ w437 _ _ _ _ _ w1008 _ _]
          tunnel: [_ w438 _ _ _ _ _ _ _ _] -> w301
          tunnel: [_ _ w493 _ _ _ _ _ _ _] -> w302
          tunnel: [_ _ w508 _ _ _ _ _ _ _] -> w300
          tunnel: [_ _ w506 _ _ _ _ _ _ _] -> w299
          tunnel: [_ _ _ _ w760 _ _ _ _ _] -> w277
          tunnel: w295 -> [_ _ _ _ _ w870 _ _ _ _]
          tunnel: w296 -> [_ _ _ _ _ w871 _ _ _ _]
          tunnel: w294 -> [_ _ _ w687 _ _ _ _ _ _]
          tunnel: [_ _ _ w682 _ _ _ _ _ _] -> w279
          tunnel: w292 -> [_ w431 _ _ _ _ _ _ _ _]
          tunnel: w291 -> [_ w430 _ _ _ _ _ w1007 _ _]
          tunnel: [_ w426 _ _ _ _ _ _ _ _] -> w290
          tunnel: [_ _ _ _ _ w869 _ _ _ _] -> w281
          tunnel: [_ _ _ _ _ w868 _ _ _ _] -> w283
          tunnel: w289 -> [_ w410 _ _ _ _ _ w995 _ _]
          tunnel: [_ w405 _ _ _ _ _ _ _ _] -> w288
          tunnel: [_ _ _ _ _ _ _ _ w1032 _] -> w266
          tunnel: w265 -> [_ _ _ _ _ _ _ _ w1026 _]
          tunnel: [_ _ _ _ _ _ _ _ w1024 _] -> w264
          tunnel: w262 -> [_ _ _ _ _ _ _ _ _ w1103]
          tunnel: [_ _ _ _ _ _ _ _ _ w1102] -> w261
          tunnel: w260 -> [_ w402 _ _ _ _ _ _ _ _]
          tunnel: [_ w397 _ _ _ _ _ _ _ _] -> w259
          tunnel: w258 -> [_ _ w487 _ _ _ _ _ _ _]
          frame #0 {
            # "Temp input channels\ninside detector"
            # "CAEN channel names\nupdater, real-time"
            # "Creates items in the menu rings, for the channel selectors on the phase diagrams;\nAlters the T warning lights."
            # "Also, dumping ground for variables and controls that may be updated during run-time"
            # "CAEN needle gauges\nMin. and Max. ranges"
            # "To view documentation of modules, look for icons that have a \"Descr.\" label near them,\nright-click these and select \"Description and tip\". For example on frame 2, \"High Voltage\",\na \"Quotient and Remainder\" icon on the left-hand side may be checked out, to view the\ndocumentation for the \"Reading Voltages and Currents\" module, which uses that icon."
            # "Time to wait, in between cycles"
            # "If the program is stopped, a final cycle executes without delay."
            # "Waiting for \"interval time\" to have passed, to start new cycle"
            n70 = Increment(x=w336) -> (x+1=w335:i32)
            "Cycle number" <- w335
            n71 = call "Is Value Changed.vim"("value"="Channel Names (CAEN)") -> ("changed or first call?"=w325:bool)
            n72 = call "Is Value Changed.vim"("value"="Specify up to six temperature sensors inside \nthe detector, separated with a comma.\nNumbers only, single commas!") -> ("changed or first call?"=w327:bool)
            n73 = case shown="True" w325 {
              tunnel: "Channel Names (CAEN)" -> [_ w342]
              frame False {
              }
              frame True {
                n74 = Index Array(array=w342) -> (element #1=→"CAEN 1.0":string, element #2=→"CAEN 1.1":string, element #3=→"CAEN 1.2":string, element #4=→"CAEN 1.3":string, element #5=→"CAEN 2.0":string, element #6=→"CAEN 2.1":string, element #7=→"CAEN 2.2 2":string, element #8=→"CAEN 2.3 2":string)  [unwired: 8 in]
                "CAEN Ch. Names" <- w342
                "Channel Names" <- w342
                "Channel Names" <- w342
              }
            }
            n75 = case shown="True" w327 {
              tunnel: "Specify up to six temperature sensors inside \nthe detector, separated with a comma.\nNumbers only, single commas!" -> [_ w352]
              frame False {
              }
              frame True {
                n76 = Bundle("Average", 666) -> (w358:cluster{string, i32})  [unwired: 1 in]
                n77 = Spreadsheet String To Array(delimiter (Tab)=",", format string="%s", spreadsheet string=w352, array type (2D Dbl)=string[] []) -> (array=w361:string[])
                n78 = for {
                  tunnel: w361 -> [w373] mode=indexing
                  tunnel: [w371] -> w360 mode=indexing
                  tunnel: [w370] -> w351 mode=indexing
                  tunnel: [w369] -> w362 mode=indexing
                  n79 = call <vilib>:"Trim Whitespace.vi"("string"=w373) -> ("trimmed string"=w369:string)  [unwired: 1 in]
                  n80 = Scan From String(input string=w369, default 1=0) -> (output 1=w370:i32)  [unwired: 3 in, 3 out]
                  n81 = Bundle("trimmed string"=w369, w370) -> (w371:cluster{"trimmed string":string, i32})  [unwired: 1 in]
                }
                "Det. T." <- w351
                n82 = Build Array (concatenate)(w360, w358) -> (w359:cluster{"trimmed string":string, i32}[])
                n83 = property on="Temperature channel selector" class="Ring (strict)"("StringsAndValues[]"=w359) -> ()  [unwired: 2 in, 2 out]
                n84 = property on="Temperature Channel Selector" class="Ring (strict)"("StringsAndValues[]"=w359) -> ()  [unwired: 2 in, 2 out]
                n85 = Index Array(array=w362) -> (element #1=→"String":string, element #2=→"String 2":string, element #3=→"String 3":string, element #4=→"String 4":string, element #5=→"String 5":string, element #6=→"String 6":string)  [unwired: 6 in]
                n86 = property on="Temperature Channel Selector" class="Ring (strict)"("StringsAndValues[]"=w360) -> ()  [unwired: 2 in, 2 out]
              }
            }
            n87 = local read "Channel Names (9207, ai0:7)"() -> (w323:string[])
            n88 = To Long Integer(number="Detector pressure input:") -> (32bit integer=→"Det.P input #":i32)
            n89 = To Long Integer(number="Flow meter input:") -> (32bit integer=→"Flow input #":i32)
            n90 = call "Is Value Changed.vim"("value"=w323) -> ("changed or first call?"=w324:bool)
            n91 = case shown="True" w324 {
              tunnel: w323 -> [_ w338]
              frame False {
                # ":D"
              }
              frame True {
                n92 = for {
                  tunnel: w338 -> [w341] mode=indexing
                  tunnel: [w339] -> w337 mode=indexing
                  i -> [w340]
                  n93 = Bundle("Or give name if \"Other\""=w341, w340) -> (w339:cluster{"Or give name if \"Other\"":string, i32})  [unwired: 1 in]
                }
                n94 = property on="Detector pressure input:" class="Ring (strict)"("StringsAndValues[]"=w337) -> ()  [unwired: 2 in, 2 out]
                n95 = property on="Flow meter input:" class="Ring (strict)"("StringsAndValues[]"=w337) -> ()  [unwired: 2 in, 2 out]
              }
            }
            n96 = case shown="False" w334 {
              tunnel: "Time per cycle (s)" -> [w390 _]
              frame False {
                n97 = while {
                  tunnel: w390 -> [w392]
                  stop <- w394 stop-if-true
                  n98 = call "Elapsed Time"("Time Target (s)"=w392) -> ("Elapsed Time (s)"=w393:dbl, "Time has Elapsed"=w394:bool)  [unwired: 11 in, 6 out]
                  n99 = Subtract(x=w392, y=w393) -> (x-y=→"Time until next cycle":dbl)
                }
              }
              frame True {
              }
            }
            n100 = stacked-sequence {
              frame #0 {
                n101 = property on="CAEN 1.0" class="Knob (strict)"("Scale.Minimum"="Scale.Range:Minimum", "Scale.Maximum"="Scale.Range:Maximum") -> ()  [unwired: 2 in, 2 out]
                n102 = property on="CAEN 1.1" class="Knob (strict)"("Scale.Minimum"="Scale.Range:Minimum 2", "Scale.Maximum"="Scale.Range:Maximum 2") -> ()  [unwired: 2 in, 2 out]
              }
              frame #1 {
                n103 = property on="CAEN 1.2" class="Knob (strict)"("Scale.Minimum"="Scale.Range:Minimum 3", "Scale.Maximum"="Scale.Range:Maximum 3") -> ()  [unwired: 2 in, 2 out]
                n104 = property on="CAEN 1.3" class="Knob (strict)"("Scale.Maximum"="Scale.Range:Maximum 4", "Scale.Minimum"="Scale.Range:Minimum 4") -> ()  [unwired: 2 in, 2 out]
              }
              frame #2 {
                n105 = property on="CAEN 2.1" class="Knob (strict)"("Scale.Maximum"="Scale.Range:Maximum 6", "Scale.Minimum"="Scale.Range:Minimum 6") -> ()  [unwired: 2 in, 2 out]
                n106 = property on="CAEN 2.0" class="Knob (strict)"("Scale.Maximum"="Scale.Range:Maximum 5", "Scale.Minimum"="Scale.Range:Minimum 5") -> ()  [unwired: 2 in, 2 out]
              }
              frame #3 {
                n107 = property on="CAEN 2.2" class="Knob (strict)"("Scale.Maximum"="Scale.Range:Maximum 7", "Scale.Minimum"="Scale.Range:Minimum 7") -> ()  [unwired: 2 in, 2 out]
                n108 = property on="CAEN 2.3" class="Knob (strict)"("Scale.Maximum"="Scale.Range:Maximum 8", "Scale.Minimum"="Scale.Range:Minimum 8") -> ()  [unwired: 2 in, 2 out]
              }
            }
          }
          frame #1 {
            # "DAQmx Read above will replace dummy data below,\nonce the 9216 modules are functioning"
            # "Descr"
            # "NI 9207 8x V, 8x mA"
            # "Case to ignore runtime errors; unpack later"
            # "Module 1 tasks+status"
            # "Temps (NI)"
            # "9216 T     (NI) x16\n9207 V     (NI)  x8\n9207 mA (NI)  x8\nTemp        (LS)  x2\nHeater %           x1"
            # "Temp A, Temp B, heater power"
            # "Measurements and conversions"
            n109 = case shown="False" "Run lakeshore?" {
              tunnel: [w461 w472] -> w438
              tunnel: w437 -> [w461 w471]
              tunnel: [-273.0 ("Input A") w470] -> w434
              tunnel: [-273.0 ("Input B") w469] -> w433
              tunnel: [73.0 ("Heater 1 (%)") w468] -> w432
              tunnel: w431 -> [_ w466]
              tunnel: [-274.0 "Setpoint (°C)"] -> w428
              frame False {
                # "Dummy data"
              }
              frame True {
                # "LS output"
                # "P\nI\nD"
                n110 = Select(t=0, s=w466, f="Heater range") -> (s? t:f=w463:i32)
                n111 = Unbundle("PID settings") -> ("P"=w477:dbl, "I"=w476:dbl, "D"=w475:dbl)
                n112 = Unbundle(w471) -> ("VISA resource name out"=w479:refnum<visa-resource-name>, "error out"=w478:errorcluster)
                n113 = call "Lakeshore subVI.vi"("Setpoint"="Setpoint (°C)", "Rate (D) (X.X %)"=w475, "Range"=w463, "Reset (I) (XX.X)"=w476, "Gain (P) (XX.X)"=w477, "error in (no error)"=w478, "VISA resource name"=w479) -> ("Input B"=w469:dbl, "Input A"=w470:dbl, "error out"=w473:errorcluster, "VISA resource name out"=w474:refnum<visa-resource-name>, "Heater 1 (%)"=w468:dbl)
                "Lakeshore" <- w473
                n114 = Bundle("VISA resource name out"=w474, "error out"=w473) -> (w472:T5)  [unwired: 1 in]
              }
            }
            n115 = Get Date/Time In Seconds() -> (seconds since 1Jan1904=w436:timestamp)
            n116 = Quotient & Remainder(x=w424, y="Read T every N cycles") -> (x-y*floor(x/y)=w427:i32)  [unwired: 1 out]
            n117 = Unbundle(w410) -> ("task out"=w409:refnum<k21>, "error out"=w408:errorcluster)
            n118 = Build Array (concatenate)(w403, w436) -> (w435:timestamp[])
            n119 = Unbundle(w430) -> ("task out"=w415:refnum<k21>, "error out"=w414:errorcluster)
            n120 = case shown="1, Default" w427 {
              tunnel: w425 -> [_ w454]
              tunnel: [w447 w450] -> w395
              tunnel: w424 -> [w446 _]
              frame 0 {
                # "Dummy data"
                # "New temperatures"
                n121 = Add(x=w446, y=-95.0 ("element")) -> (x+y=w449:dbl)
                n122 = Initialize Array(w449, 16) -> (w447:dbl[])
              }
              frame 1, Default {
                # "Gets 1st 16 Col's\nfrom last row:\nPrevious 16 temps."
                # "Get previous temps"
                n123 = Array Size(array=w454) -> (size(s)=w456:i32[])
                n124 = Index Array(array=w456, index=0) -> (element=w457:i32)
                n125 = Decrement(x=w457) -> (x-1=w453:i32)
                n126 = Index Array(array=w454, index (row)=w453) -> (element=w452:dbl[])  [unwired: 1 in]
                n127 = Array Subset(array=w452, length=16) -> (w450:dbl[])  [unwired: 1 in]
              }
            }
            n128 = call-poly <vilib>:"DAQmx Read.vi"("task/channels in"=w409, "error in"=w408) -> ("task out"=w407:refnum<k21>, "data"=→"PT100 data":dbl[], "error out"=w406:errorcluster)  [unwired: 11 in]
            "NI 9216 x2" <- w406
            n129 = call-poly <vilib>:"DAQmx Read.vi"("task/channels in"=w415, "error in"=w414) -> ("task out"=w413:refnum<k21>, "data"=w422:dbl[], "error out"=w412:errorcluster)  [unwired: 11 in]
            "Raw readouts (V, mA)" <- w422
            "NI 9207" <- w412
            n130 = Build Array (concatenate)("Offsets\nsubtracted", "Offsets\nsubtracted") -> (w416:dbl[])
            n131 = Build Array (concatenate)("Multipliers", "Multipliers") -> (w419:dbl[])
            n132 = for {
              tunnel: w416 -> [w444] mode=indexing
              tunnel: w422 -> [w443] mode=indexing
              tunnel: w419 -> [w441] mode=indexing
              tunnel: [w440] -> w423 mode=indexing
              n133 = Subtract(x=w443, y=w444) -> (x-y=w442:dbl)
              n134 = Multiply(x=w442, y=w441) -> (x*y=w440:dbl)
            }
            n135 = Bundle("task out"=w407, "error out"=w406) -> (w405:T4)  [unwired: 1 in]
            n136 = Bundle("task out"=w413, "error out"=w412) -> (w426:T4)  [unwired: 1 in]
            n137 = Build Array(w434, w433, w432) -> (w411:dbl[])
            "LakeShore readings" <- w411
            n138 = Unbundle(w402) -> ("task out"=w401:refnum<k21>, "error out"=w400:errorcluster)
            n139 = call-poly <vilib>:"DAQmx Read.vi"("task/channels in"=w401, "error in"=w400) -> ("task out"=w399:refnum<k21>, "data"=w396:dbl[], "error out"=w398:errorcluster)  [unwired: 11 in]
            "NI 9226" <- w398
            "PT1000 data" <- w396
            n140 = Bundle("task out"=w399, "error out"=w398) -> (w397:T4)  [unwired: 1 in]
          }
          frame #2 {
            # "Alter voltages if button clicked"
            # "2"
            # "1"
            # "Descr."
            # "Descr."
            # "VMON1  x4 \nVMON2  x4\nIMON1    x4\nIMON2    x4"
            # "Needle gauge Voltage displays"
            # "1"
            # "2"
            # "1"
            # "2"
            # "Reads new V and A every N cycles,\nor passes previous values"
            # "High Voltage"
            n141 = Quotient & Remainder(x=w518, y="Read CAEN units \nevery N cycles") -> (x-y*floor(x/y)=w497:i32)  [unwired: 1 out]
            n142 = Unbundle(w525) -> ("VISA resource name out"=w489:refnum<visa-resource-name>, "error out"=w524:errorcluster)
            n143 = Unbundle(w522) -> ("VISA resource name out"=w488:refnum<visa-resource-name>, "error out"=w521:errorcluster)
            n144 = Build Array (concatenate)("VSet (V)", "VMax (V)", "IMax (uA)") -> (w502:dbl[])
            n145 = case shown="0" w497 {
              tunnel: w489 -> [w666 _]
              tunnel: w524 -> [w665 w677]
              tunnel: w523 -> [_ w673]
              tunnel: w488 -> [w659 _]
              tunnel: w521 -> [w656 w678]
              tunnel: [w655 w678] -> w483
              tunnel: [w662 w677] -> w486
              tunnel: [w648 w673] -> w493
              tunnel: [w650 w674] -> w520
              tunnel: [w649 w670] -> w519
              tunnel: w487 -> [w651 _]
              frame 0 {
                # "All data x16"
                # "Voltages x8"
                # "Currents x8"
                # "Read"
                n146 = call "READ_SUPPLY.vi"("VISA resource name"=w666, "Board address"=u8 0, "NChannels"=u8 4, "error in (no error)"=w665) -> ("VMon values (V)"=w661:dbl[], "IMon values (uA)"=w660:dbl[], "error out"=w662:errorcluster)  [unwired: 9 in]
                n147 = call "READ_SUPPLY.vi"("VISA resource name"=w659, "Board address"=u8 0, "NChannels"=u8 4, "error in (no error)"=w656) -> ("VMon values (V)"=w654:dbl[], "IMon values (uA)"=w653:dbl[], "error out"=w655:errorcluster)  [unwired: 9 in]
                n148 = Build Array (concatenate)(w661, w654) -> (w652:dbl[])
                n149 = Build Array (concatenate)(w660, w653) -> (w649:dbl[])
                n150 = for {
                  tunnel: w652 -> [w668] mode=indexing
                  tunnel: w651 -> [w669] mode=indexing
                  tunnel: [w667] -> w650 mode=indexing
                  n151 = Multiply(x=w669, y=w668) -> (x*y=w667:dbl)
                }
                n152 = Build Array (concatenate)(w650, w649) -> (w648:dbl[])
              }
              frame 1, Default {
                # "Don't read: pass previous"
                n153 = Array Subset(array=w673, index=0, length=8) -> (w674:dbl[])
                n154 = Array Subset(array=w673, index=8, length=8) -> (w670:dbl[])
              }
            }
            "Voltages" <- w520
            "Vmon (V)" <- w520
            "IMon (uA)" <- w519
            n155 = Build Array("Apply Voltage", "Set to zero", "Kill voltage") -> (w496:bool[])
            n156 = case shown="True" "Query HV status" {
              tunnel: w489 -> [_ w537]
              tunnel: w488 -> [_ w536]
              tunnel: w483 -> [w526 w531]
              tunnel: w486 -> [w527 w530]
              tunnel: [w527 w529] -> w491
              tunnel: [w526 w528] -> w490
              frame False {
              }
              frame True {
                w539 = u8 0 ("Board address")
                w538 = u8 4 ("NChannels")
                n157 = Bundle("VISA resource name out"=w537, "Board address"=w539, "NChannels"=w538) -> (w534:T6)  [unwired: 1 in]
                n158 = Bundle("VISA resource name out"=w536, "Board address"=w539, "NChannels"=w538) -> (w535:T6)  [unwired: 1 in]
                n159 = call <instrlib>:"Channel Status.vi"("error in (no error)"=w530, "BoardHandle"=w534) -> ("error out"=w529:errorcluster, "Channel Status Array"=→"CAEN 1":T2)  [unwired: 7 in, 1 out]
                n160 = call <instrlib>:"Channel Status.vi"("error in (no error)"=w531, "BoardHandle"=w535) -> ("error out"=w528:errorcluster, "Channel Status Array"=→"CAEN 2":T2)  [unwired: 7 in, 1 out]
              }
            }
            n161 = Search 1D Array(1D array=w496, element=TRUE) -> (index of element=w510:i32)  [unwired: 1 in]
            n162 = case shown="0" w510 {
              tunnel: w489 -> [w553 w588 w621 w647]
              tunnel: w488 -> [w543 w580 w612 w646]
              tunnel: [w554 w589 w622 w645] -> w485
              tunnel: [w553 w588 w621 w647] -> w509
              tunnel: [w542 w579 w611 w644] -> w482
              tunnel: [w543 w580 w612 w646] -> w507
              tunnel: "VSet (V)" -> [w551 _ w619 _]
              tunnel: "VMax (V)" -> [w550 w586 _ _]
              tunnel: "IMax (uA)" -> [w549 w585 w618 _]
              tunnel: w491 -> [w541 w578 w610 w645]
              tunnel: w490 -> [w540 w577 w609 w644]
              frame 0 {
                w544 = 4 ("length")
                w548 = 4 ("length")
                # "Last four"
                # "First four"
                # "Apply voltage"
                n163 = Array Subset(array=w551, length=w548) -> (w556:dbl[])  [unwired: 1 in]
                n164 = Array Subset(array=w550, length=w548) -> (w555:dbl[])  [unwired: 1 in]
                n165 = Array Subset(array=w549, length=w548) -> (w552:dbl[])  [unwired: 1 in]
                n166 = Array Subset(array=w551, index=w544) -> (w547:dbl[])  [unwired: 1 in]
                n167 = Array Subset(array=w550, index=w544) -> (w546:dbl[])  [unwired: 1 in]
                n168 = Array Subset(array=w549, index=w544) -> (w545:dbl[])  [unwired: 1 in]
                n169 = for {
                  tunnel: w553 -> [w575]
                  tunnel: w541 -> [w574]
                  tunnel: w556 -> [w571] mode=indexing
                  tunnel: w555 -> [w569] mode=indexing
                  tunnel: w552 -> [w568] mode=indexing
                  tunnel: [w567] -> w554
                  i -> [w576]
                  n170 = call "SET_SUPPLY_CHANNEL.vi"("VISA resource name"=w575, "Voltage Level (0.0 V)"=w571, "Enable (OFF)"=TRUE, "Board address"=u8 0, "NChannels"=u8 4, "Channel (0)"=w576, "error in (no error)"=w574, "Voltage Max (0.0 V)"=w569, "Current Limit (0.00 uA)"=w568) -> ("error out"=w567:errorcluster)  [unwired: 6 in]
                }
                n171 = for {
                  tunnel: w543 -> [w566]
                  tunnel: w540 -> [w560]
                  tunnel: w547 -> [w565] mode=indexing
                  tunnel: w546 -> [w564] mode=indexing
                  tunnel: w545 -> [w563] mode=indexing
                  tunnel: [w559] -> w542
                  i -> [w562]
                  n172 = call "SET_SUPPLY_CHANNEL.vi"("VISA resource name"=w566, "Voltage Level (0.0 V)"=w565, "Enable (OFF)"=TRUE, "Board address"=u8 0, "NChannels"=u8 4, "Channel (0)"=w562, "error in (no error)"=w560, "Voltage Max (0.0 V)"=w564, "Current Limit (0.00 uA)"=w563) -> ("error out"=w559:errorcluster)  [unwired: 6 in]
                }
              }
              frame 1 {
                w581 = 4 ("length")
                w584 = 4 ("length")
                # "Set V to zero"
                n173 = Array Subset(array=w585, length=w584) -> (w587:dbl[])  [unwired: 1 in]
                n174 = Array Subset(array=w586, length=w584) -> (w590:dbl[])  [unwired: 1 in]
                n175 = Array Subset(array=w586, index=w581) -> (w583:dbl[])  [unwired: 1 in]
                n176 = Array Subset(array=w585, index=w581) -> (w582:dbl[])  [unwired: 1 in]
                n177 = for {
                  tunnel: w588 -> [w607]
                  tunnel: w578 -> [w606]
                  tunnel: w590 -> [w603] mode=indexing
                  tunnel: w587 -> [w602] mode=indexing
                  tunnel: [w601] -> w589
                  i -> [w608]
                  w600 = u8 0 ("Board address")
                  n178 = call "SET_SUPPLY_CHANNEL.vi"("VISA resource name"=w607, "Voltage Level (0.0 V)"=w600, "Enable (OFF)"=TRUE, "Board address"=w600, "NChannels"=u8 4, "Channel (0)"=w608, "error in (no error)"=w606, "Voltage Max (0.0 V)"=w603, "Current Limit (0.00 uA)"=w602) -> ("error out"=w601:errorcluster)  [unwired: 6 in]
                }
                n179 = for {
                  tunnel: w580 -> [w591]
                  tunnel: w577 -> [w596]
                  tunnel: w583 -> [w595] mode=indexing
                  tunnel: w582 -> [w594] mode=indexing
                  tunnel: [w592] -> w579
                  i -> [w597]
                  w599 = 0 ("length")
                  n180 = call "SET_SUPPLY_CHANNEL.vi"("VISA resource name"=w591, "Voltage Level (0.0 V)"=w599, "Enable (OFF)"=TRUE, "Board address"=w599, "NChannels"=u8 4, "Channel (0)"=w597, "error in (no error)"=w596, "Voltage Max (0.0 V)"=w595, "Current Limit (0.00 uA)"=w594) -> ("error out"=w592:errorcluster)  [unwired: 6 in]
                }
              }
              frame 2 {
                w613 = 4 ("length")
                w616 = 2 ("length")
                w617 = 4 ("length")
                # "CAEN 2: Top gate, Bottom gate"
                # "CAEN 1 values:\nPMT1&2, Anode, Cathode"
                # "Set VMax to zero, \"Kill\""
                n181 = Array Subset(array=w618, length=w617) -> (w620:dbl[])  [unwired: 1 in]
                n182 = Array Subset(array=w619, length=w617) -> (w623:dbl[])  [unwired: 1 in]
                n183 = Array Subset(array=w619, index=w613, length=w616) -> (w615:dbl[])
                n184 = Array Subset(array=w618, index=w613, length=w616) -> (w614:dbl[])
                n185 = for {
                  tunnel: w621 -> [w642]
                  tunnel: w610 -> [w641]
                  tunnel: w623 -> [w638] mode=indexing
                  tunnel: w620 -> [w636] mode=indexing
                  tunnel: [w635] -> w622
                  i -> [w643]
                  n186 = call "SET_SUPPLY_CHANNEL.vi"("VISA resource name"=w642, "Voltage Level (0.0 V)"=w638, "Enable (OFF)"=TRUE, "Board address"=u8 0, "NChannels"=u8 4, "Channel (0)"=w643, "error in (no error)"=w641, "Voltage Max (0.0 V)"=u8 0 ("Board address"), "Current Limit (0.00 uA)"=w636) -> ("error out"=w635:errorcluster)  [unwired: 6 in]
                }
                n187 = for {
                  tunnel: w612 -> [w624]
                  tunnel: w609 -> [w627]
                  tunnel: w615 -> [w630] mode=indexing
                  tunnel: w614 -> [w628] mode=indexing
                  tunnel: [w626] -> w611
                  i -> [w633]
                  n188 = call "SET_SUPPLY_CHANNEL.vi"("VISA resource name"=w624, "Voltage Level (0.0 V)"=w630, "Enable (OFF)"=TRUE, "Board address"=u8 0, "NChannels"=u8 4, "Channel (0)"=w633, "error in (no error)"=w627, "Voltage Max (0.0 V)"=0, "Current Limit (0.00 uA)"=w628) -> ("error out"=w626:errorcluster)  [unwired: 6 in]
                }
              }
              frame 3, Default {
                # "\"Executes\" if none of the three buttons have been clicked"
                # "Do nothing"
              }
            }
            n189 = Merge Errors(w486, w485) -> (→"CAEN 1":errorcluster)
            n190 = Bundle("VISA resource name out"=w509, "error out"=w485) -> (w508:T5)  [unwired: 1 in]
            n191 = Bundle("VISA resource name out"=w507, "error out"=w482) -> (w506:T5)  [unwired: 1 in]
            n192 = Merge Errors(w483, w482) -> (→"CAEN 2":errorcluster)
            n193 = Index Array(array=w493) -> (element #1=→"CAEN 1.0":dbl, element #2=→"CAEN 1.1":dbl, element #3=→"CAEN 1.2":dbl, element #4=→"CAEN 1.3":dbl, element #5=→"CAEN 2.0":dbl, element #6=→"CAEN 2.1":dbl, element #7=→"CAEN 2.2":dbl, element #8=→"CAEN 2.3":dbl)  [unwired: 8 in]
          }
          frame #3 {
            # "Descr."
            # "Reset anode"
            n194 = Or Array Elements(Boolean array=w680) -> (logical OR=w679:bool)
            n195 = case shown="True" "Reset anode\nperiodically?" {
              tunnel: w687 -> [_ w693]
              tunnel: w686 -> [_ w702]
              tunnel: w685 -> [_ w707]
              tunnel: w679 -> [_ w691]
              tunnel: [w688 w692] -> w682
              tunnel: w681 -> [_ w701]
              frame False {
                # "Anode Reset Routine inactive:\nkeep timers up to date so activating\nroutine will correctly initiate the timers."
                n196 = Get Date/Time In Seconds() -> (seconds since 1Jan1904=w690:timestamp)
                n197 = To Double Precision Float(number=w690) -> (double precision float=w689:dbl)
                n198 = Build Array(w689, w689) -> (w688:dbl[])
              }
              frame True {
                # "Descr."
                n199 = case shown="\"CAEN 1\", Default" "CAEN unit selector" {
                  tunnel: w702 -> [w721 _]
                  tunnel: w701 -> [_ w723]
                  tunnel: [w721 w723] -> w700
                  tunnel: [0 4] -> w698
                  frame "CAEN 1", Default {
                  }
                  frame "CAEN 2" {
                  }
                }
                n200 = call "anode_timing.vi"("Keep off for X seconds"="Keep off for X seconds", "Array of timers"=w693, "Kill every Y minutes"="Kill every Y minutes") -> ("Time to kill"=w709:bool, "Time until reset"=→"Seconds until \nanode reset":dbl, "Time until autokill"=→"Seconds until \nanode autokill":dbl, "Time to reset"=w710:bool)  [unwired: 5 in]
                "Killed" <- w709
                "Restarted" <- w710
                n201 = Add(x=w698, y="Anode ch.") -> (x+y=w696:i32)
                n202 = Build Array(w709, w710, w691) -> (w713:bool[])
                n203 = Add(x=w696, y=8) -> (x+y=w703:i32)
                n204 = Add(x=w696, y=16) -> (x+y=w704:i32)
                n205 = Search 1D Array(1D array=w713, element=TRUE) -> (index of element=w712:i32)  [unwired: 1 in]
                n206 = Unbundle(w700) -> ("VISA resource name out"=w718:refnum<visa-resource-name>, "error out"=w717:errorcluster)
                n207 = Index Array(array=w707, index #1=w696, index #2=w703, index #3=w704) -> (element #1=w716:dbl, element #2=w714:dbl, element #3=w715:dbl)
                n208 = case shown="2" w712 {
                  tunnel: w716 -> [_ w747 _ _]
                  tunnel: w714 -> [w732 w746 _ _]
                  tunnel: w715 -> [w734 w745 _ _]
                  tunnel: w718 -> [w739 w750 _ _]
                  tunnel: w717 -> [w738 w749 _ _]
                  tunnel: "Anode ch." -> [w730 w743 _ _]
                  tunnel: w693 -> [w725 _ _ w756]
                  tunnel: [w724 w740 w753 w756] -> w692
                  frame 0 {
                    # "Set Anode Voltage to zero,\nreset the 1st timer"
                    # "Anode Vset to zero"
                    n209 = Get Date/Time In Seconds() -> (seconds since 1Jan1904=w728:timestamp)
                    n210 = Index Array(array=w725, index=1) -> (element=w726:dbl)
                    n211 = To Double Precision Float(number=w728) -> (double precision float=w727:dbl)
                    n212 = call "SET_SUPPLY_CHANNEL.vi"("VISA resource name"=w739, "Voltage Level (0.0 V)"=0.0, "Enable (OFF)"=TRUE, "Board address"=u8 0, "NChannels"=u8 4, "Channel (0)"=w730, "error in (no error)"=w738, "Voltage Max (0.0 V)"=w732, "Current Limit (0.00 uA)"=w734) -> ("error out"=w733:errorcluster)  [unwired: 6 in]
                    n213 = Build Array(w727, w726) -> (w724:dbl[])
                    n214 = call <vilib>:"Simple Error Handler.vi"("error in (no error)"=w733) -> ()  [unwired: 4 in, 5 out]
                  }
                  frame 1 {
                    # "Set Anode Voltage to defined value,\nreset both timers"
                    # "Anode Vset applied"
                    n215 = Get Date/Time In Seconds() -> (seconds since 1Jan1904=w742:timestamp)
                    n216 = To Double Precision Float(number=w742) -> (double precision float=w741:dbl)
                    n217 = call "SET_SUPPLY_CHANNEL.vi"("VISA resource name"=w750, "Voltage Level (0.0 V)"=w747, "Enable (OFF)"=TRUE, "Board address"=u8 0, "NChannels"=u8 4, "Channel (0)"=w743, "error in (no error)"=w749, "Voltage Max (0.0 V)"=w746, "Current Limit (0.00 uA)"=w745) -> ("error out"=w744:errorcluster)  [unwired: 6 in]
                    n218 = Build Array(w741, w741) -> (w740:dbl[])
                    n219 = call <vilib>:"Simple Error Handler.vi"("error in (no error)"=w744) -> ()  [unwired: 4 in, 5 out]
                  }
                  frame 2 {
                    # "Change Voltage button pressed"
                    # "Reset both timers"
                    n220 = Get Date/Time In Seconds() -> (seconds since 1Jan1904=w755:timestamp)
                    n221 = To Double Precision Float(number=w755) -> (double precision float=w754:dbl)
                    n222 = Build Array(w754, w754) -> (w753:dbl[])
                  }
                  frame 3, Default {
                    # "Timers stay at previous value,\nso difference between those and\ncurrent time keeps incrementing"
                    # "No event"
                  }
                }
              }
            }
            n223 = To Time Stamp(1:w682) -> (0:→"Anode timers":timestamp[])
            "?" <- "Reset anode\nperiodically?"
          }
          frame #4 {
            # "Flexibly acquire indices"
            # "Plots 9207 output vs time"
            # "Descr."
            # "Moving averages"
            # "Historic graphs: Phase, 9207 ai, Flow, Heater, Temperature"
            # "Non-historic Temperature + Det. Pressure"
            # "Updated TOBA"
            # "Descr."
            # "Latest Detector Pressure"
            # "Plots individual lists of Temp. vs. t"
            # "Plots and moving averages"
            n224 = Build Array (concatenate)(w772, w770, w767, w771) -> (w803:dbl[])
            n225 = Build Array (concatenate)(w804, w803) -> (w758:dbl[][])
            "TOBA appended" <- w758
            n226 = Array Size(array=w767) -> (size(s)=w766:i32)
            n227 = Array Size(array=w770) -> (size(s)=w768:i32)
            n228 = Array Size(array=w772) -> (size(s)=w769:i32)
            n229 = Add(x=w769, y=w768) -> (x+y=w757:i32)
            n230 = Add(x=w757, y=w766) -> (x+y=w765:i32)
            n231 = local read "Det. T."() -> (w782:i32[])
            n232 = local read "Flow input #"() -> (w778:i32)
            n233 = local read "Det.P input #"() -> (w779:i32)
            n234 = Equal?(x=666, y="Temperature channel selector") -> (x = y?=w797:bool)
            n235 = Add(x=w765, y=2 ("disabled index (col)")) -> (x+y=w763:i32)
            n236 = case shown="True" w797 {
              tunnel: w772 -> [w835 w841]
              tunnel: w782 -> [_ w840]
              tunnel: [w834 w836] -> w795
              tunnel: "Temperature channel selector" -> [w833 _]
              frame False {
                n237 = Index Array(array=w835, index=w833) -> (element=w834:dbl)
              }
              frame True {
                n238 = for {
                  tunnel: w841 -> [w844]
                  tunnel: w840 -> [w843] mode=indexing
                  tunnel: [w842] -> w837 mode=indexing
                  n239 = Index Array(array=w844, index=w843) -> (element=w842:dbl)
                }
                n240 = Array Size(array=w837) -> (size(s)=w839:i32)
                n241 = Add Array Elements(numeric array=w837) -> (sum=w838:dbl)
                n242 = Divide(x=w838, y=w839) -> (x/y=w836:dbl)
              }
            }
            n243 = Add(x=w779, y=w757) -> (x+y=w790:i32)
            n244 = Add(x=w757, y=w778) -> (x+y=w788:i32)
            n245 = Index Array(array=w758, index (col)=w763) -> (element=w761:dbl[])  [unwired: 1 in]
            n246 = Index Array(array=w758, index (col)="Temperature Channel Selector") -> (element=w793:dbl[])  [unwired: 1 in]
            n247 = Index Array(array=w758, index (col) #1=w790, index (col) #2=w788) -> (element #1=w789:dbl[], element #2=w776:dbl[])  [unwired: 2 in]
            n248 = local read "Det.P input #"() -> (w780:i32)
            n249 = Bundle(w760, w761) -> (w762:cluster{timestamp[], dbl[]})  [unwired: 1 in]
            n250 = Bundle(w793, w789) -> (w808:cluster{dbl[], dbl[]})  [unwired: 1 in]
            n251 = for {
              N: 8 -> [_]
              tunnel: w758 -> [w826]
              tunnel: w760 -> [w819]
              tunnel: [w823] -> w786 mode=indexing
              tunnel: [w818] -> w785 mode=indexing
              tunnel: w757 -> [w816]
              i -> [w822]
              n252 = Add(x=w816, y=8) -> (x+y=w815:i32)
              n253 = Add(x=w816, y=w822) -> (x+y=w825:i32)
              n254 = Add(x=w822, y=w815) -> (x+y=w821:i32)
              n255 = Index Array(array=w826, index (col) #1=w825, index (col) #2=w821) -> (element #1=w824:dbl[], element #2=w820:dbl[])  [unwired: 2 in]
              n256 = Bundle(w819, w824) -> (w823:cluster{timestamp[], dbl[]})  [unwired: 1 in]
              n257 = Bundle(w819, w820) -> (w818:cluster{timestamp[], dbl[]})  [unwired: 1 in]
            }
            "9207 (ai 0:7, Volts)" <- w786
            "9207 (ai 8:15, Amperes)" <- w785
            n258 = Build Array(w762) -> (→"Heater power (%)":cluster{timestamp[], dbl[]}[])
            n259 = Bundle(w760, w776) -> (w806:cluster{timestamp[], dbl[]})  [unwired: 1 in]
            n260 = Build Array(w808) -> (→"Historical Large Phase Diagram":cluster{dbl[], dbl[]}[])
            n261 = Index Array(array=w767, index=w780) -> (element=w809:dbl)
            n262 = Build Array(w806) -> (→"Flow (SLPM)":cluster{timestamp[], dbl[]}[])
            n263 = call "moving_avg.vi"("N samples"="N samples", "Array"=w789) -> ("Numeric"=→"Detector Pressure":dbl)  [unwired: 9 in]
            n264 = call "moving_avg.vi"("N samples"="N samples", "Array"=w776) -> ("Numeric"=→"Average Flow (SLPM)":dbl)  [unwired: 9 in]
            n265 = Bundle(w795, w809) -> (w813:cluster{dbl, dbl})  [unwired: 1 in]
            n266 = Build Array(w813) -> (→"Phase Diagram":cluster{dbl, dbl}[])
            n267 = local read "Det. T."() -> (w781:i32[])
            n268 = Equal?(x=666, y="Temperature Channel Selector") -> (x = y?=w799:bool)
            n269 = for {
              N: w757 -> [_]
              tunnel: w760 -> [w861]
              tunnel: [w860] -> w814 mode=indexing
              tunnel: w758 -> [w859]
              i -> [w858]
              n270 = Index Array(array=w859, index (col)=w858) -> (element=w857:dbl[])  [unwired: 1 in]
              n271 = Bundle(w861, w857) -> (w860:cluster{timestamp[], dbl[]})  [unwired: 1 in]
            }
            "Temperature (ai 0:15, °C)" <- w814
            n272 = case shown="True" w799 {
              tunnel: w772 -> [w847 w853]
              tunnel: w781 -> [_ w852]
              tunnel: [w846 w848] -> w802
              tunnel: "Temperature Channel Selector" -> [w845 _]
              frame False {
                n273 = Index Array(array=w847, index=w845) -> (element=w846:dbl)
              }
              frame True {
                n274 = for {
                  tunnel: w853 -> [w856]
                  tunnel: w852 -> [w855] mode=indexing
                  tunnel: [w854] -> w849 mode=indexing
                  n275 = Index Array(array=w856, index=w855) -> (element=w854:dbl)
                }
                n276 = Array Size(array=w849) -> (size(s)=w851:i32)
                n277 = Add Array Elements(numeric array=w849) -> (sum=w850:dbl)
                n278 = Divide(x=w850, y=w851) -> (x/y=w848:dbl)
              }
            }
            n279 = local read "Channel Names (9207, ai8:15)"() -> (w784:string[])
            n280 = local read "Channel Names (9207, ai0:7)"() -> (w783:string[])
            n281 = call "Is Value Changed.vim"("value"=w784) -> ("changed or first call?"=w791:bool)
            n282 = call "Is Value Changed.vim"("value"=w783) -> ("changed or first call?"=w792:bool)
            n283 = case shown="True" w791 {
              tunnel: w784 -> [_ w827]
              frame False {
              }
              frame True {
                n284 = for {
                  tunnel: w827 -> [w828] mode=indexing
                  i -> [w829]
                  n285 = property on="9207 (ai 8:15, Amperes)" class="XYGraph (strict)"("Active Plot"=w829, "Plot.Plot Name"=w828) -> ()  [unwired: 2 in, 2 out]
                }
              }
            }
            n286 = Bundle(w802, w809) -> (w811:cluster{dbl, dbl})  [unwired: 1 in]
            n287 = case shown="True" w792 {
              tunnel: w783 -> [_ w830]
              frame False {
              }
              frame True {
                n288 = for {
                  tunnel: w830 -> [w831] mode=indexing
                  i -> [w832]
                  n289 = property on="9207 (ai 0:7, Volts)" class="XYGraph (strict)"("Active Plot"=w832, "Plot.Plot Name"=w831) -> ()  [unwired: 2 in, 2 out]
                }
              }
            }
            n290 = Build Array(w811) -> (→"Large Phase Diagram":cluster{dbl, dbl}[])
          }
          frame #5 {
            # "Temp A, Temp B, Heater%"
            # "Temperatures x16\nTo indicators on the physical schematic"
            # "Individual latest 9207 readings.\nIndicators go here. Array is 1x16,\nitems have been converted using\nthe offsets and multipliers"
            # "Displays"
            n291 = local read "Flow input #"() -> (w865:i32)
            n292 = case shown="False" "Reset?" {
              tunnel: [w877 0.0] -> w873
              tunnel: w870 -> [w877 _]
              frame False {
              }
              frame True {
              }
            }
            n293 = Index Array(array=w864) -> ()  [unwired: 16 in, 16 out]
            n294 = Index Array(array=w864, index=w865) -> (element=w868:dbl)
            n295 = call "Average_flow_x_time.vi"("Array of timestamps"=w872, "Previous Flow"=w871, "Latest Flow"=w868) -> ("Volume (SL)"=w874:dbl)  [unwired: 8 in]
            n296 = case shown="False" "Pause?" {
              tunnel: w873 -> [w881 w882]
              tunnel: w874 -> [w880 _]
              tunnel: [w879 w882] -> w869
              frame False {
                n297 = Add(x=w880, y=w881) -> (x+y=w879:dbl)
              }
              frame True {
              }
            }
            "Integrated Flow (SL)" <- w869
            n298 = Index Array(array=w866) -> (element #1=→"Coldhead" →"Temp A":dbl, element #2=→"Heater" →"Temp B":dbl)  [unwired: 3 in, 1 out]
            n299 = Index Array(array=w867) -> ()  [unwired: 16 in, 16 out]
            "9207 (V; A) Converted" <- w864
            "9216 #1 (°C)" <- w867
            "9216 #2 (°C)" <- w867
          }
          frame #6 {
            # "The same order applies to the headers re-saved,\nbut with an additional line, stating the date/time"
            # "-----------DATA SAVED----------\nHuman-readable timestamp  ;\nTemperatures (16),  2xNI 9216;\nVolts, Amps  (8 x2),     NI 9207;\nTemperature (2),    Lakeshore;\nHeater power (1),  Lakeshore;\nSetpoint (1),           Lakeshore;\nHV readouts (16)          CAEN ;\nCurrent time (s)                ---   ;\nCycle time (s)                    ---   ;"
            # "Saving data"
            n300 = Get Date/Time In Seconds() -> (seconds since 1Jan1904=w904:timestamp)
            n301 = To Double Precision Float(number=w904) -> (double precision float=w890:dbl)
            n302 = Build Array (concatenate)(w885, w893, w892, w905, w891, w890, w889) -> (w903:dbl[])
            n303 = Array Size(array=w885) -> (size(s)=w886:i32)
            n304 = Array Size(array=w884) -> (size(s)=w887:i32)
            n305 = Add(x=w886, y=w887) -> (x+y=w883:i32)
            n306 = Get Date/Time String() -> (date string=w897:string)  [unwired: 3 in, 1 out]
            n307 = case shown="True" "Re-save headers" {
              tunnel: w883 -> [_ w906]
              frame False {
                # "Just sit around and feel pretty"
              }
              frame True {
                w914 = ""
                # "Append line of most recent channel names to header file"
                n308 = local read "Channel Names (CAEN)"() -> (w913:string[])
                n309 = local read "Channel Names (9207, ai0:7)"() -> (w921:string[])
                n310 = for {
                  N: w906 -> [_]
                  shift-right: [w945] -> w917
                  shift-left: "" -> [w946]
                  i -> [w950]
                  n311 = Format Into String(initial string="t", w950) -> (resulting string=w948:string)  [unwired: 2 in, 1 out]
                  n312 = Concatenate Strings(w946, w948, "\t") -> (w945:string)
                }
                n313 = for {
                  shift-right: [w943] -> w919
                  shift-left: w914 -> [w944]
                  tunnel: w921 -> [w941] mode=indexing
                  n314 = Concatenate Strings(w944, w941, "\t") -> (w943:string)
                }
                n315 = local read "Channel Names (9207, ai8:15)"() -> (w920:string[])
                n316 = for {
                  tunnel: w913 -> [w935] mode=indexing
                  shift-right: [w933] -> w908
                  shift-left: w914 -> [w932]
                  n317 = Concatenate Strings(w932, w935, " (V)", "\t") -> (w933:string)
                }
                n318 = for {
                  shift-right: [w939] -> w916
                  shift-left: w919 -> [w940]
                  tunnel: w920 -> [w937] mode=indexing
                  n319 = Concatenate Strings(w940, w937, "\t") -> (w939:string)
                }
                n320 = for {
                  tunnel: w913 -> [w930] mode=indexing
                  shift-right: [w928] -> w912
                  shift-left: w908 -> [w927]
                  n321 = Concatenate Strings(w927, w930, " (I)", "\t") -> (w928:string)
                }
                n322 = Get Date/Time String() -> (date string=w925:string)  [unwired: 3 in, 1 out]
                n323 = Format Date/Time String() -> (date/time string=w907:string)  [unwired: 3 in]
                n324 = Build Path(base path=path "D:/Log_data/SC_LOG_HEADERS", name or relative path=w925) -> (appended path=w924:path)
                n325 = Concatenate Strings("Time\t", w917, w916, "Temp A\tTemp B\tHeater Power\tSetpoint\t", w912, "Time in seconds\tTime per cycle\t", w907, "\r\n") -> (w909:string)
                n326 = call <vilib>:"Write Spreadsheet String.vi"("append to file? (new file:F)"=TRUE, "spreadsheet string"=w909, "file path (dialog if empty)"=w924) -> ()  [unwired: 7 in, 2 out]
              }
            }
            n327 = Build Path(base path=path "D:/Log_data/SC_LOG", name or relative path=w897) -> (appended path=w896:path)
            n328 = Format Date/Time String() -> (date/time string=w901:string)  [unwired: 3 in]
            n329 = Array To Spreadsheet String(array=w903, 3:"%.3f" ("format string")) -> (spreadsheet string=w899:string)  [unwired: 1 in]
            n330 = Concatenate Strings(w901, "\t", w899) -> (w895:string)
            n331 = call <vilib>:"Write Spreadsheet String.vi"("append to file? (new file:F)"=TRUE, "spreadsheet string"=w895, "file path (dialog if empty)"=w896) -> ()  [unwired: 7 in, 2 out]
          }
          frame #7 {
            # "Status is True if ANY (armed)\ncondition is met"
            # "Detector P. Alert"
            # "Uninteruptable\n Power Supply Alert"
            # "Temp. Warning"
            # "Arms"
            # "Comm. Alert"
            # "Temperature Alert"
            # "Alarm conditions (Temp)"
            # "Check Alarms and Warnings"
            n332 = Unbundle By Name(w995) -> ("error out.status"=w976:bool)
            "NI mod 2&3 status" <- w976
            n333 = Unbundle By Name(w1008) -> ("error out.status"=w1006:bool)
            "LakeShore status" <- w1006
            n334 = Unbundle By Name(w1010) -> ("error out.status"=w1005:bool)
            "CAEN 1 status" <- w1005
            n335 = Unbundle By Name(w1009) -> ("error out.status"=w1004:bool)
            "CAEN 2 status" <- w1004
            n336 = Unbundle By Name(w1007) -> ("error out.status"=w1003:bool)
            "NI mod1 (P) status" <- w1003
            n337 = Build Array(w1006, w1005, w1004, w1003, w976) -> (w977:bool[])
            n338 = Build Array("LakeShore", "CAEN 1", "CAEN 2", "NI mod 2&3", "NI mod 1") -> (w972:bool[])
            n339 = call "check_ups.vi"() -> ("Error: no voltages read"=w956:bool, "Timestamp last measured"=→"Timestamp last \nmeasured (UPS)":timestamp, "Minimum input voltage measured"=w966:dbl)  [unwired: 8 in, 1 out]
            "Minimum input voltage measured" <- w966
            n340 = property on="Det.P input #" class="DigNum (strict)"() -> ("Value"=w992:i32)  [unwired: 2 in, 2 out]
            n341 = Or Array Elements(Boolean array=w977) -> (logical OR=→"Comm. status":bool)
            n342 = for {
              tunnel: w977 -> [w1013] mode=indexing
              tunnel: w972 -> [w1012] mode=indexing
              tunnel: [w1011] -> w971 mode=indexing
              n343 = And(x=w1013, y=w1012) -> (x .and. y?=w1011:bool)
            }
            n344 = Index Array(array=w993, index=w992) -> (element=w989:dbl)
            n345 = Less?(x=w966, y="UPS Voltage \nLower Threshold") -> (x < y?=w958:bool)
            n346 = Equal?(x=w966, y=-1.0) -> (x = y?=w957:bool)
            n347 = Less?(x=w989, y="Underpressure threshold") -> (x < y?=w987:bool)
            n348 = Build Array(w958, w957, w956) -> (w955:bool[])
            n349 = Or Array Elements(Boolean array=w971) -> (logical OR=w961:bool)
            n350 = Greater?(x=w989, y="Overpressure threshold") -> (0:w988:bool)
            n351 = Or(x=w988, y=w987) -> (x .or. y?=w986:bool)
            "Det. P. warning" <- w986
            n352 = Or Array Elements(Boolean array=w955) -> (logical OR=w954:bool)
            "Warning" <- w954
            n353 = And(x="UPS", y=w954) -> (x .and. y?=w960:bool)
            n354 = And(x=w986, y="Detector Pressure") -> (x .and. y?=w962:bool)
            n355 = local read "Det. T."() -> (w952:i32[])
            n356 = Build Array("T 1", "T 2", "T 3", "T 4", "T 5", "T 6") -> (w951:bool[])
            n357 = for {
              tunnel: w994 -> [w1023]
              tunnel: w952 -> [w1022] mode=indexing
              tunnel: w951 -> [w1016] mode=indexing
              tunnel: [w1015] -> w963 mode=indexing
              tunnel: [w1014] -> w978 mode=indexing
              n358 = Index Array(array=w1023, index=w1022) -> (element=w1019:dbl)
              n359 = Less?(x=w1019, y="Low Temp threshold") -> (x < y?=w1018:bool)
              n360 = Greater?(x=w1019, y="High Temp threshold") -> (0:w1017:bool)
              n361 = Or(x=w1018, y=w1017) -> (x .or. y?=w1014:bool)
              n362 = And(x=w1016, y=w1014) -> (x .and. y?=w1015:bool)
            }
            n363 = Index Array(array=w978) -> (element #1=→"Boolean":bool, element #2=→"Boolean 2":bool, element #3=→"Boolean 3":bool, element #4=→"Boolean 4":bool, element #5=→"Boolean 5":bool, element #6=→"Boolean 6":bool)  [unwired: 6 in]
            n364 = Build Array (concatenate)(w963, w962, w961, w960) -> (w959:bool[])
            n365 = Or Array Elements(Boolean array=w959) -> (logical OR=w953:bool)
            "Alarm state" <- w953
          }
          frame #8 {
            # "Testing alarm will not interfere"
            # "Act on alarm"
            n366 = Or(x="Test alarm", y=w1030) -> (x .or. y?=w1031:bool)
            n367 = case shown="True" w1031 {
              tunnel: "Test alarm" -> [_ w1038]
              tunnel: w1028 -> [_ w1046]
              tunnel: w1027 -> [_ w1045]
              tunnel: w1026 -> [w1034 w1036]
              tunnel: "Alarm\nMaster switch" -> [_ w1043]
              tunnel: [w1034 w1037] -> w1024
              frame False {
                # "Timer stays at previous value"
              }
              frame True {
                n368 = Get Date/Time In Seconds() -> (seconds since 1Jan1904=w1050:timestamp)
                n369 = case shown="True" "\"Sound\" alarm" {
                  frame False {
                  }
                  frame True {
                    n370 = call <vilib>:"Beep.vi"("duration (msec)"=u32 1000, "frequency (Hz)"="Sound alarm\nFrequency (Hz)") -> ()  [unwired: 10 in]
                  }
                }
                n371 = To Double Precision Float(number=w1050) -> (double precision float=w1047:dbl)
                n372 = Multiply(x="Repeat Alarm SMS\nevery N minutes", y=60.0) -> (x*y=w1039:dbl)
                n373 = Subtract(x=w1047, y=w1036) -> (x-y=w1042:dbl)
                n374 = Greater?(x=w1042, y=w1039) -> (0:w1044:bool)
                n375 = And(x=w1043, y=w1044) -> (x .and. y?=w1041:bool)
                n376 = Or(x=w1038, y=w1041) -> (x .or. y?=w1040:bool)
                n377 = case shown="True" w1040 {
                  tunnel: w1038 -> [_ w1065]
                  tunnel: w1046 -> [_ w1073]
                  tunnel: w1045 -> [_ w1061]
                  tunnel: [w1053 w1063] -> w1037
                  tunnel: w1036 -> [w1053 w1062]
                  frame False {
                    # "Alarm not armed, or defined time has not yet passed"
                  }
                  frame True {
                    # "Average T in Det."
                    n378 = local read "Det. T."() -> (w1079:i32[])
                    n379 = local read "Det.P input #"() -> (w1080:i32)
                    n380 = case shown="True" w1065 {
                      tunnel: ["Error encountered inXAMS! Status:" "TESTING the XAMS alarm. Status:"] -> w1072
                      tunnel: [w1084 w1087] -> w1063
                      tunnel: w1062 -> [_ w1087]
                      frame False {
                        n381 = Get Date/Time In Seconds() -> (seconds since 1Jan1904=w1085:timestamp)
                        n382 = To Double Precision Float(number=w1085) -> (double precision float=w1084:dbl)
                      }
                      frame True {
                      }
                    }
                    n383 = for {
                      tunnel: w1061 -> [w1098]
                      tunnel: w1079 -> [w1094] mode=indexing
                      tunnel: [w1097] -> w1078 mode=indexing
                      tunnel: [w1095] -> w1056 mode=indexing
                      n384 = Index Array(array=w1098, index=w1094) -> (element=w1097:dbl)
                      n385 = Format Into String(format string="%.0f", w1094) -> (resulting string=w1092:string)  [unwired: 2 in, 1 out]
                      n386 = Format Into String(format string="%.1f", w1097) -> (resulting string=w1090:string)  [unwired: 2 in, 1 out]
                      n387 = Concatenate Strings("\n" ("format string"), w1092, "     " ("format string"), w1090) -> (w1095:string)
                    }
                    n388 = Index Array(array=w1073, index=w1080) -> (element=w1074:dbl)
                    n389 = Array Size(array=w1078) -> (size(s)=w1076:i32)
                    n390 = Add Array Elements(numeric array=w1078) -> (sum=w1077:dbl)
                    n391 = Format Into String(format string="%.3f", w1074) -> (resulting string=w1068:string)  [unwired: 2 in, 1 out]
                    n392 = Divide(x=w1077, y=w1076) -> (x/y=w1066:dbl)
                    n393 = Format Date/Time String() -> (date/time string=w1070:string)  [unwired: 3 in]
                    n394 = Format Into String(format string="%.2f", w1066) -> (resulting string=w1054:string)  [unwired: 2 in, 1 out]
                    n395 = Concatenate Strings(w1072, "\nDate/time: ", w1070, "\nDetector Pressure: ", w1068, " bar", "\nDetector Temperatures (°C):", "\nCh:   Temp:" ("format string"), w1056, "\nAverage detector temperature: ", w1054) -> (w1060:string)
                    "Alarm (or test) message" <- w1060
                    n396 = for {
                      tunnel: w1060 -> [w1083]
                      tunnel: "Phone numbers" -> [w1082] mode=indexing
                      n397 = call "send_sms.vi"("Message content"=w1083, "Phone number"=w1082) -> ("standard error"=→"SMS error":string)  [unwired: 8 in, 1 out]
                    }
                  }
                }
              }
            }
            n398 = And(x="Shut off heater \nif Alarm is active", y=w1030) -> (x .and. y?=w1032:bool)
            "Alarm active 2" <- "Alarm\nMaster switch"
          }
          frame #9 {
            # "Daily e-mail"
            n399 = Get Date/Time In Seconds() -> (seconds since 1Jan1904=w1111:timestamp)
            n400 = To Double Precision Float(number=w1111) -> (double precision float=w1110:dbl)
            n401 = Get Date/Time String(want seconds? (F)=FALSE) -> (time string=w1113:string)  [unwired: 2 in, 1 out]
            n402 = Subtract(x=w1110, y=w1103) -> (x-y=w1109:dbl)
            n403 = Equal?(x=w1113, y="Send status email at time:") -> (x = y?=w1106:bool)
            n404 = Greater?(x=w1109, y=62) -> (0:w1105:bool)
            n405 = Build Array("Send daily email?", w1106, w1105) -> (w1104:bool[])
            n406 = And Array Elements(Boolean array=w1104) -> (logical AND=w1100:bool)
            n407 = Or(x="Send status email now", y=w1100) -> (x .or. y?=w1101:bool)
            n408 = case shown="True" w1101 {
              tunnel: w1117 -> [_ w1152]
              tunnel: w1116 -> [_ w1135]
              tunnel: w1115 -> [_ w1144]
              tunnel: w1103 -> [w1118 _]
              tunnel: [w1118 w1130] -> w1102
              frame False {
              }
              frame True {
                # "Average T in Det."
                n409 = local read "Det. T."() -> (w1153:i32[])
                n410 = Not Equal To 0?(x="Number of Bonus lines") -> (x != 0?=w1123:bool)
                n411 = case shown="True" w1123 {
                  tunnel: [w1158 w1161] -> w1124
                  tunnel: "Number of Bonus lines" -> [_ w1164]
                  frame False {
                    n412 = Build Array("\n[Flavor text module inactive]") -> (w1158:string[])
                  }
                  frame True {
                    n413 = Build Path(base path=path "C:/Users/xams/Desktop/New XAMS Slow Control", name or relative path="cool_beans.txt") -> (appended path=w1165:path)
                    n414 = call-poly <vilib>:"Read Delimited Spreadsheet.vi"("file path (dialog if empty)"=w1165) -> ("all rows"=w1168:string[][])  [unwired: 9 in, 5 out]
                    n415 = Array Size(array=w1168) -> (size(s)=w1170:i32[])
                    n416 = Index Array(array=w1170) -> (element=w1169:i32)  [unwired: 1 in]
                    n417 = for {
                      N: w1164 -> [_]
                      tunnel: w1169 -> [w1175]
                      tunnel: w1168 -> [w1174]
                      tunnel: [w1171] -> w1162 mode=indexing
                      n418 = Random Number (0-1)() -> (number: 0 to 1=w1178:dbl)
                      n419 = Multiply(x=w1175, y=w1178) -> (x*y=w1177:dbl)
                      n420 = Round To Nearest(number=w1177) -> (nearest integer value=w1176:dbl)
                      n421 = Index Array(array=w1174, index (row)=w1176) -> (element=w1172:string[])  [unwired: 1 in]
                      n422 = Concatenate Strings("\n", w1172) -> (w1171:string)
                    }
                    n423 = Concatenate Strings("\n\nCool beans of the day: ", w1162) -> (w1160:string)
                    n424 = Build Array(w1160) -> (w1161:string[])
                  }
                }
                n425 = local read "Det.P input #"() -> (w1145:i32)
                n426 = for {
                  tunnel: w1153 -> [w1187] mode=indexing
                  tunnel: [w1188] -> w1137 mode=indexing
                  tunnel: w1152 -> [w1181]
                  tunnel: [w1180] -> w1151 mode=indexing
                  n427 = Index Array(array=w1181, index=w1187) -> (element=w1180:dbl)
                  n428 = Format Into String(format string="%.0f", w1187) -> (resulting string=w1184:string)  [unwired: 2 in, 1 out]
                  n429 = Format Into String(format string="%.2f", w1180) -> (resulting string=w1182:string)  [unwired: 2 in, 1 out]
                  n430 = Concatenate Strings("\nCh: " ("format string"), w1184, ", Temp: " ("format string"), w1182, "°C." ("format string")) -> (w1188:string)
                }
                n431 = Array Size(array=w1151) -> (size(s)=w1156:i32)
                n432 = Add Array Elements(numeric array=w1151) -> (sum=w1157:dbl)
                n433 = Index Array(array=w1144, index=w1145) -> (element=w1142:dbl)
                n434 = Divide(x=w1157, y=w1156) -> (x/y=w1154:dbl)
                n435 = Format Into String(format string="%.3f", w1142) -> (resulting string=w1140:string)  [unwired: 2 in, 1 out]
                n436 = Format Into String(format string="%.2f", w1154) -> (resulting string=w1134:string)  [unwired: 2 in, 1 out]
                n437 = Select(t="ACTIVE!!!!!", s=w1135, f="inactive.") -> (s? t:f=w1147:string)
                n438 = Concatenate Strings("Hello, XAMS teammembers.", "\n\nThe alarm is currently ", w1147, "\n\nThe latest detector pressure is: ", w1140, " bar." ("format string"), "\nTemperatures inside the detector are:", w1137, "\nThe average detector temperature is ", w1134, "°C." ("format string"), "\n\nThank you for doing your best today, once again!\nRegards, SC.", w1124) -> (w1129:string)
                "Status email preview" <- w1129
                n439 = call "custom_email_program.vi"("mail server"="smtp.nikhef.nl", "return address"="return address", "message"=w1129, "subject ([No Subject])"="XAMS daily status email.", "Email Adresses"="Email Addresses") -> ("error out"=w1121:errorcluster)  [unwired: 6 in]
                n440 = Unbundle By Name(w1121) -> ("code"=→"Email error":i32, "source"=→"source":string)
                n441 = Get Date/Time In Seconds() -> (seconds since 1Jan1904=w1131:timestamp)
                n442 = To Double Precision Float(number=w1131) -> (double precision float=w1130:dbl)
              }
            }
          }
        }
        n443 = Decrement(x="Cycles to execute") -> (x-1=w287:dbl)
        n444 = Decrement(x=w287) -> (x-1=w286:dbl)
        n445 = Greater?(x=w270, y=w286) -> ()  [unwired: 1 out]
        n446 = Decrement(x="Clear data every N cycles") -> (x-1=w267:dbl)
        n447 = Greater?(x=w270, y=w267) -> (0:w269:bool)
        n448 = And(x="Auto-clear data?", y=w269) -> (x .and. y?=w272:bool)
        n449 = Or(x=w272, y="Clear data") -> (x .or. y?=w274:bool)
        n450 = case shown="False" w274 {
          tunnel: w285 -> [w315 _]
          tunnel: [w315 dbl[][] []] -> w284
          tunnel: w283 -> [w314 _]
          tunnel: [w314 w321] -> w282
          tunnel: w281 -> [w313 _]
          tunnel: [w313 w321] -> w280
          tunnel: w279 -> [w312 _]
          tunnel: [w312 w319] -> w278
          tunnel: w277 -> [w311 _]
          tunnel: [w311 w317] -> w276
          tunnel: w270 -> [w310 _]
          tunnel: [w310 0] -> w271
          frame False {
          }
          frame True {
            w321 = 0.0
            n451 = Get Date/Time In Seconds() -> (seconds since 1Jan1904=w318:timestamp)
            n452 = To Double Precision Float(number=w318) -> (double precision float=w320:dbl)
            n453 = Build Array(w318) -> (w317:timestamp[])
            n454 = Build Array(w320, w320) -> (w319:dbl[])
          }
        }
        n455 = Or(x=FALSE, y="stop") -> (x .or. y?=w307:bool)
        "Auto-clear" <- "Auto-clear data?"
      }
    }
    frame True {
    }
  }
  n456 = flat-sequence {
    tunnel: w20 -> [w1232]
    tunnel: w16 -> [w1223]
    tunnel: w15 -> [w1220]
    tunnel: w14 -> [w1215]
    tunnel: w7 -> [w1204]
    tunnel: w2 -> [w1201]
    frame #0 {
      w1228 = u16 2 items=["1"=1, "2"=2] ("Heater Output (1:1)")
      w1229 = u16 0 items=["Off", "Low (On)", "Medium", "High"] ("Range (0:Off)")
      # "Important icons! Always press STOP button when done \ninstead of force closing, otherwise these don't get executed"
      # "Turn off heater, shutdown COM"
      # "Error Handling and Post-Processing (EHaPP)"
      n457 = Unbundle(w1232) -> ("VISA resource name out"=w1231:refnum<visa-resource-name>, "error out"=w1230:errorcluster)
      n458 = Unbundle(w1223) -> ("VISA resource name out"=w1222:refnum<visa-resource-name>, "error out"=w1221:errorcluster)
      n459 = Unbundle(w1220) -> ("VISA resource name out"=w1219:refnum<visa-resource-name>, "error out"=w1218:errorcluster)
      n460 = Unbundle(w1215) -> ("task out"=w1213:refnum<k21>, "error out"=w1211:errorcluster)
      n461 = Unbundle(w1204) -> ("task out"=w1208:refnum<k21>, "error out"=w1206:errorcluster)
      n462 = Unbundle(w1201) -> ("task out"=w1200:refnum<k21>, "error out"=w1199:errorcluster)
      n463 = call <vilib>:"DAQmx Stop Task.vi"("task/channels in"=w1213, "error in"=w1211) -> ("task out"=w1212:refnum<k21>, "error out"=w1210:errorcluster)  [unwired: 12 in]
      n464 = call <vilib>:"DAQmx Stop Task.vi"("task/channels in"=w1208, "error in"=w1206) -> ("task out"=w1207:refnum<k21>, "error out"=w1205:errorcluster)  [unwired: 12 in]
      n465 = call <vilib>:"DAQmx Stop Task.vi"("task/channels in"=w1200, "error in"=w1199) -> ("task out"=w1198:refnum<k21>, "error out"=w1202:errorcluster)  [unwired: 12 in]
      n466 = call <instrlib>:"Configure Output Range and Manual Value.vi"("VISA resource name"=w1231, "Heater Output (1:1)"=w1228, "Range (0:Off)"=w1229, "Manual Output (0.00 %)"=0.0, "error in (no error)"=w1230) -> ("VISA resource name out"=w1226:refnum<visa-resource-name>, "error out"=w1225:errorcluster)  [unwired: 9 in]
      n467 = call <instrlib>:"Close.vi"("error in (no error)"=w1221, "VISA resource name"=w1222) -> ("error out"=w1217:errorcluster)  [unwired: 9 in]
      n468 = call <instrlib>:"Close.vi"("error in (no error)"=w1218, "VISA resource name"=w1219) -> ("error out"=w1216:errorcluster)  [unwired: 9 in]
      n469 = call <instrlib>:"Close.vi"("error in (no error)"=w1225, "VISA resource name"=w1226) -> ("error out"=w1224:errorcluster)  [unwired: 9 in]
      n470 = call <vilib>:"DAQmx Clear Task.vi"("task in"=w1212, "error in"=w1210) -> ("error out"=w1214:errorcluster)  [unwired: 13 in]
      n471 = call <vilib>:"DAQmx Clear Task.vi"("task in"=w1207, "error in"=w1205) -> ("error out"=w1209:errorcluster)  [unwired: 13 in]
      n472 = call <vilib>:"DAQmx Clear Task.vi"("task in"=w1198, "error in"=w1202) -> ("error out"=w1203:errorcluster)  [unwired: 13 in]
      n473 = call <vilib>:"Simple Error Handler.vi"("error in (no error)"=w1224) -> ()  [unwired: 4 in, 5 out]
      n474 = call <vilib>:"Simple Error Handler.vi"("error in (no error)"=w1217) -> ()  [unwired: 4 in, 5 out]
      n475 = call <vilib>:"Simple Error Handler.vi"("error in (no error)"=w1216) -> ()  [unwired: 4 in, 5 out]
      n476 = call <vilib>:"Simple Error Handler.vi"("error in (no error)"=w1214) -> ()  [unwired: 4 in, 5 out]
      n477 = call <vilib>:"Simple Error Handler.vi"("error in (no error)"=w1209) -> ()  [unwired: 4 in, 5 out]
      n478 = call <vilib>:"Simple Error Handler.vi"("error in (no error)"=w1203) -> ()  [unwired: 4 in, 5 out]
    }
  }
  n479 = Array Size(array=w30) -> (size(s)=w33:i32)
  n480 = Decrement(x=w33) -> (x-1=w32:i32)
  n481 = Index Array(array=w30, index #1=w32, index #2=1 ("index")) -> (element #1=w31:timestamp, element #2=w12:timestamp)
  n482 = To Double Precision Float(number=w31) -> (double precision float=w29:dbl)
  n483 = To Double Precision Float(number=w12) -> (double precision float=w28:dbl)
  n484 = Subtract(x=w29, y=w28) -> ()  [unwired: 1 out]
  "Started up?" <- w24
